vi "Main HMI.vi"() -> ()   [LabVIEW 2020]
uses:
  Control/State - Main HMI.ctl
  Control/Page List Configuration.ctl
  <vilib>/Utility/miscctls.llb/LVRectTypeDef.ctl
  <vilib>/Utility/miscctls.llb/LVPointTypeDef.ctl
  <vilib>/Utility/miscctls.llb/LVPositionTypeDef.ctl
  Control/State - FGV.ctl
  <vilib>/picture/picture.llb/imagedata.ctl
  Control/Header - Page.ctl
  <vilib>/Utility/miscctls.llb/LVBoundsTypeDef.ctl
  Control/State - eFGV.ctl
  Control/Header - User Management.ctl
  Control/Section.ctl
  <vilib>/Platform/browser.llb/Open URL in Default Browser (string).vi
panel:
  out "Project Name":string
  out "Version":string="v1.0"
  in  "Developer":bool
  out "Logo":picture
  in  "Acquire":bool
  out "Log Time":dbl format="%<%H:%M:%S>t"
  in  "Log":bool
  in  "Left":bool caption="1"
  in  "Page":T1(radio)=enum."2"
  in  "Right":bool caption="11"
  in  "Screenshot":bool
  in  "Info":bool
  in  "Alarm Event":bool
  in  "Logout":bool
  in  "Close":bool
  out "Disable":bool
  in  "Error in":errorcluster
  out "Error out":errorcluster
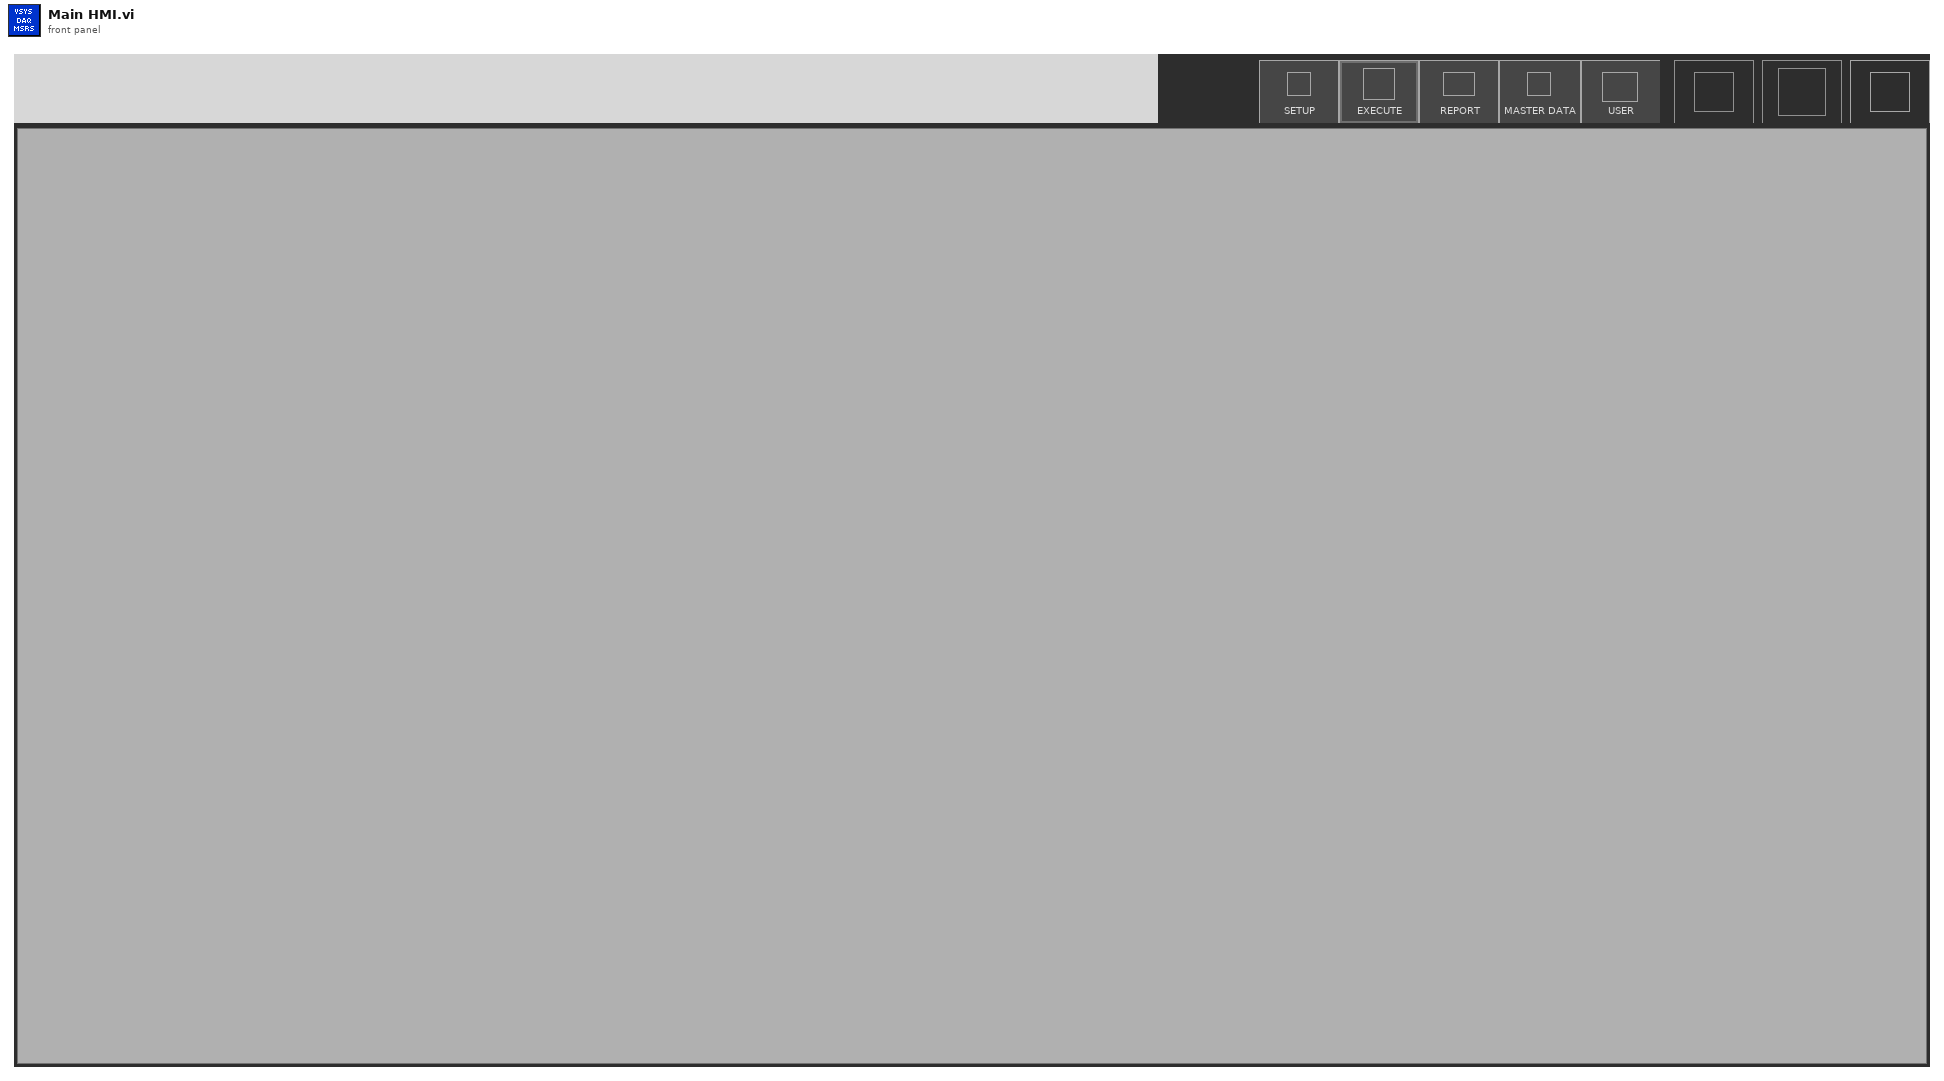
[diagram p1: front panel]
types:
  T1 = enum32{"1", "2", "3", "4", "5", "6", "7", "8", "9", "10", "11", "12", "13", "14", "15"}
  T2 = typedef "Page List Configuration.ctl" = cluster{"HMI Configuration":cluster{"EXE Name":string, "Project Name":string, "Max Page No":i32, "HMI State":enum32{"Invalid", "Standard", "Closed", "Hidden", "Minimized", "Maximized"}, "Version":enum16{"Demo", "User"}, "Check License":bool, "Font Size":u32, "Res: Height":i16, "Res: Width":i16, "License Level":enum16{"Level 1", "Level 2", "Level 3", "Level 4", "Level 5"}, "License Type":enum16{"Free", "Trial", "Subscription", "Perpetual"}}, "All HMI Module":string[], "Default HMI Module":string[], "Page Module":string[], "Page List: Level 1":string[], "Page List: Level 2":string[], "Page List: Level 3":string[], "All RT Module":string[], "Default RT Module":string[], "Acquire Enable Page":string[], "Log Enable Page":string[], "Run Page":string[], "Kill Page":string[], "Button":cluster{"Text":string[], "Tip Strip":string[]}}
  T3 = typedef "LVRectTypeDef.ctl" = cluster{"Left":i16, "Top":i16, "Right":i16, "Bottom":i16}
  T4 = cluster{"Config":T2, "Module":cluster{"Run Module":string[], "Kill Module":string[], "Page Module":string[], "Enable Page":string[]}, "Page Name":string, "T_Out":i32, "Time":timestamp, "Acquire":bool, "Log":bool, "Login":bool, "Discover":bool, "Button Ref":refnum<vi>[], "Direction":string, "Page Size":i32, "Content Area Rect":T3, "Page Size (Hidden)":i32, "Force Logout?":bool, "Update Button":bool, "Event Ref":refnum<event-registration>}
  T5 = typedef "State - Main HMI.ctl" = enum16{"Init", "Init Logo & Name", "Init Size", "Init Page", "Init Button Page", "Init Splitter", "Register Events", "Init Module", "Run Module", "Kill Module", "Change Page", "Update Button Page", "Close Splash Screen", "Idle", "Screenshot", "Developer Mode", "Info", "Move Button Page", "Acquire Event", "Log Event", "Logout", "Check for Exit", "Close"}
  T6 = typedef "LVPositionTypeDef.ctl" = cluster{"Left":i32, "Top":i32}
  T7 = typedef "State - FGV.ctl" = enum16{"Write", "Read"}
  T8 = typedef "imagedata.ctl" = cluster{"image type":i32, "image depth":i32, "image":u8[], "mask":u8[], "colors":u32[], "Rectangle":cluster{"left":i16, "top":i16, "right":i16, "bottom":i16}}
  T9 = enum16{"Init", "Init Module", "Run Module", "Kill Module", "Change Page", "Exit"}
  T10 = typedef "Header - Page.ctl" = enum16{"P1 Main", "P2", "P3 Analysis", "P4 Prediction", "P5 User"}
  T11 = enum8{"Enabled", "Disabled", "Disabled and Grayed Out"}
  T12 = typedef "LVBoundsTypeDef.ctl" = cluster{"Width":u32, "Height":u32}
  T13 = typedef "Header - User Management.ctl" = enum16{"Name", "Staff ID", "Username", "Password", "Access Level", "Status", "Access Page"}
  T14 = enum32{"Invalid", "Standard", "Closed", "Hidden", "Minimized", "Maximized"}
  T15 = enum32{"invalid app kind", "Development System", "Run Time System", "Student Edition", "Embedded LabVIEW", "Evaluation", "Custom"}
  T16 = typedef "Section.ctl" = enum16{"Software Setup", "Config", "Setup", "Network Stream", "MQTT Client", "Setting", "Sample Interval", "Calibration", "Pre-Ranging", "Overrun", "Static", "Filter", "Properties", "Alarm", "Device", "Logging"}
  T17 = typedef "LVPointTypeDef.ctl" = cluster{"Horizontal":i16, "Vertical":i16}
  T18 = typedef "State - eFGV.ctl" = enum16{"Init", "Read", "Write", "Exit"}
  T19 = typedef "License File Parameter.ctl" = cluster{"Expired Time":string, "Computer ID":string, "Product Name":string, "Period":i16, "Activated Time":string, "License Level":enum16{"Level 1", "Level 2", "Level 3", "Level 4", "Level 5"}, "License Type":enum16{"Free", "Trial", "Subscription", "Perpetual"}, "Log Time":string}
  T20 = enum16{"Free", "Trial", "Subscription", "Perpetual"}
  T21 = cluster{"Page Name":string, "All Module":string[], "Default Run Module":string[], "Page Module":string[]}
  T22 = enum16{"Level 1", "Level 2", "Level 3", "Level 4", "Level 5"}
  T23 = enum16{"Pre-Ranging", "Overrun", "Static", "Analysis", "Prediction"}
  T24 = enum32{"Bad", "Idle", "Run top level", "Running"}
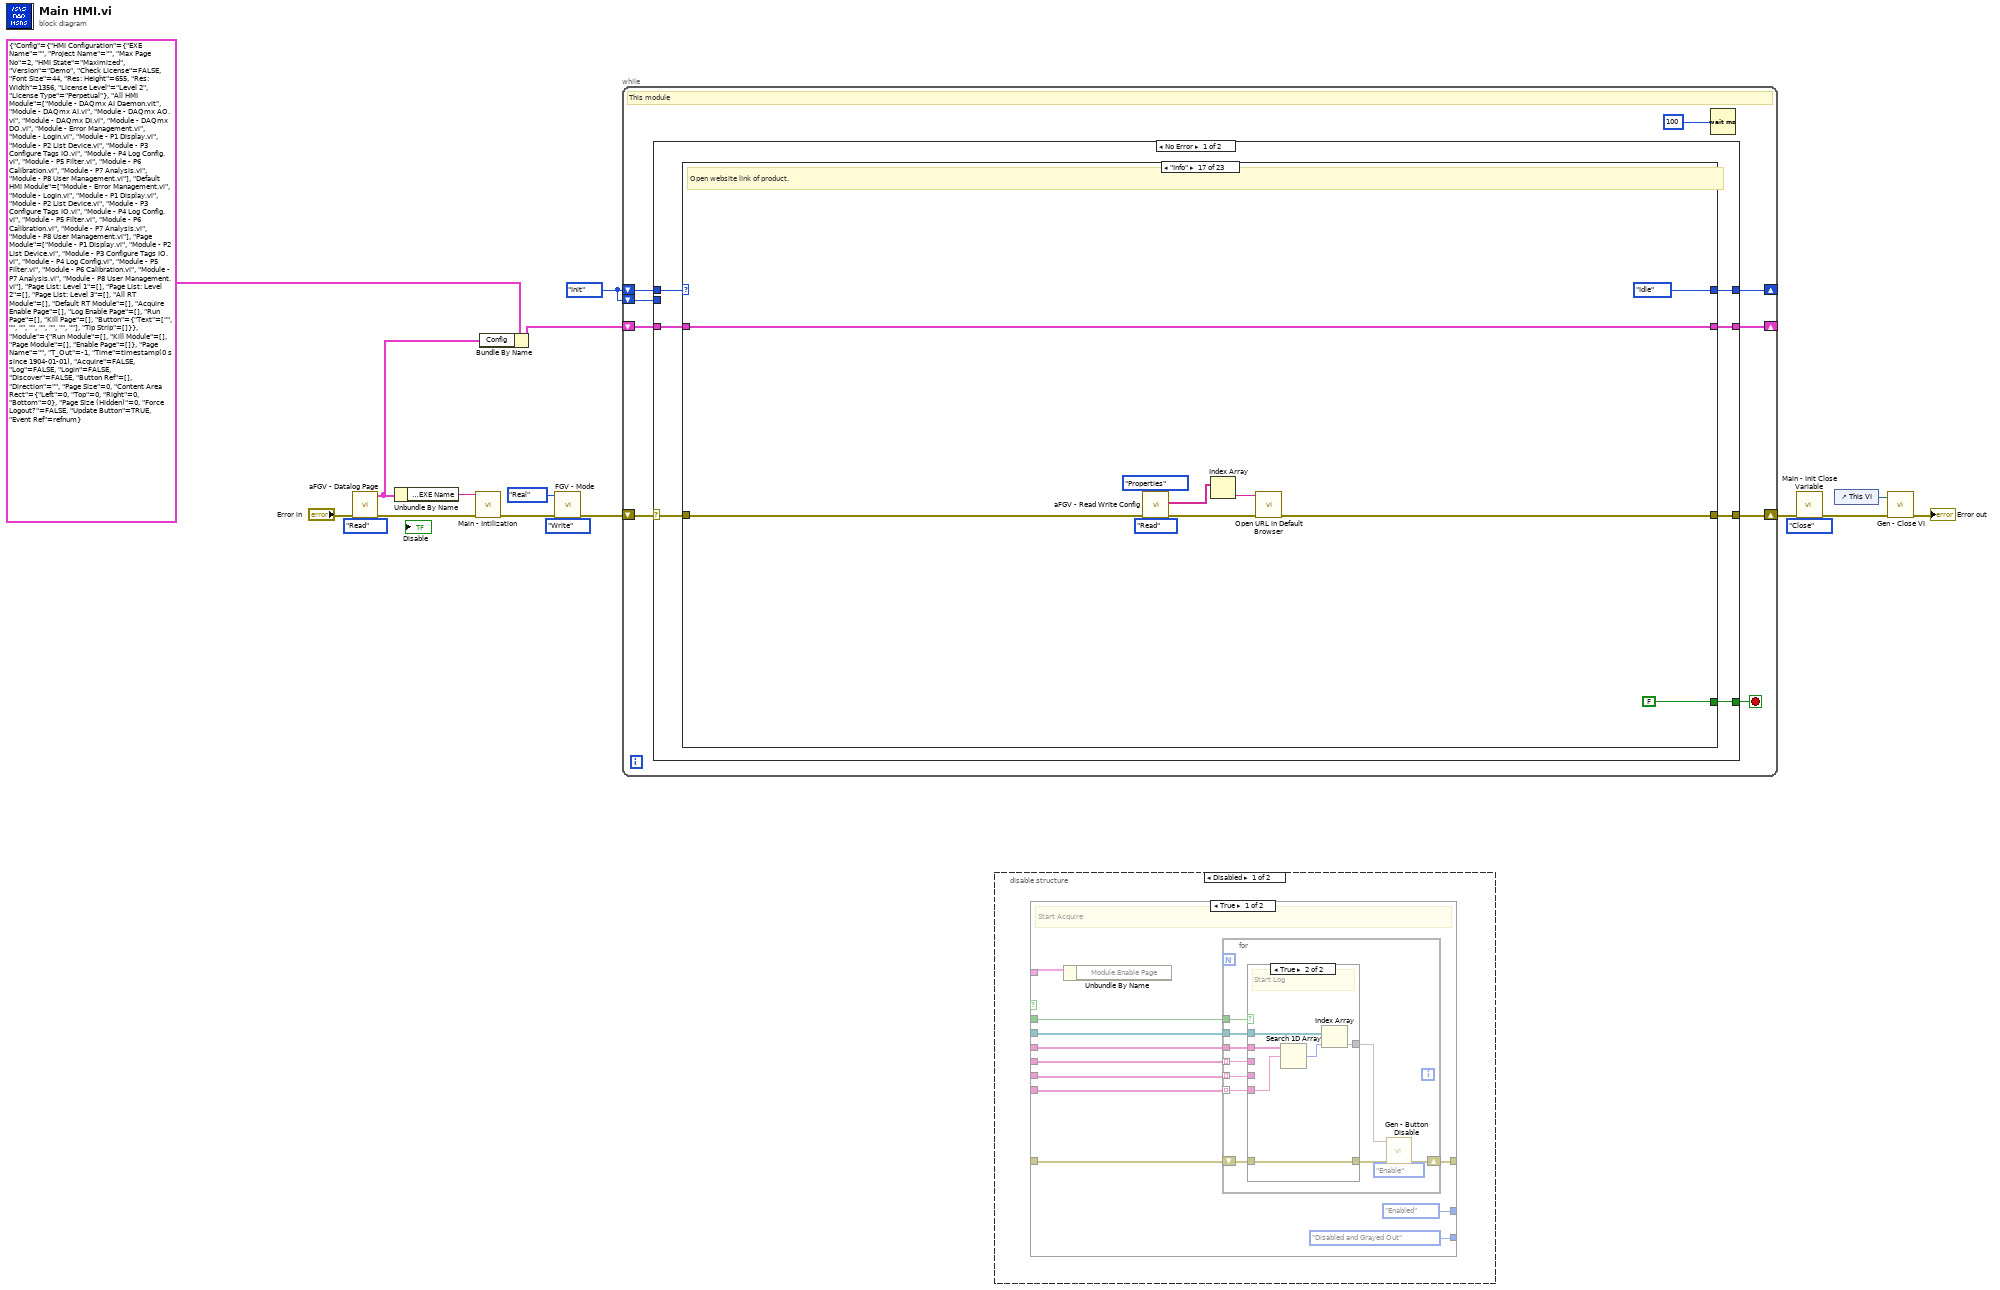
[diagram p0: block diagram]
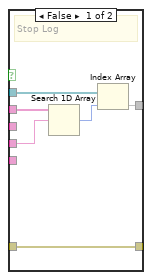
[diagram p2: hidden frame]
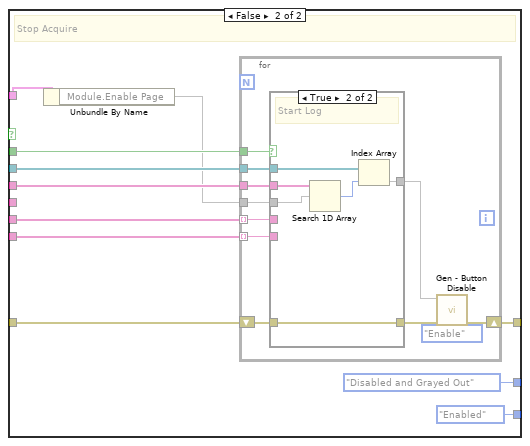
[diagram p3: hidden frame]
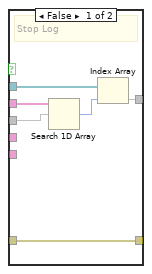
[diagram p4: hidden frame]
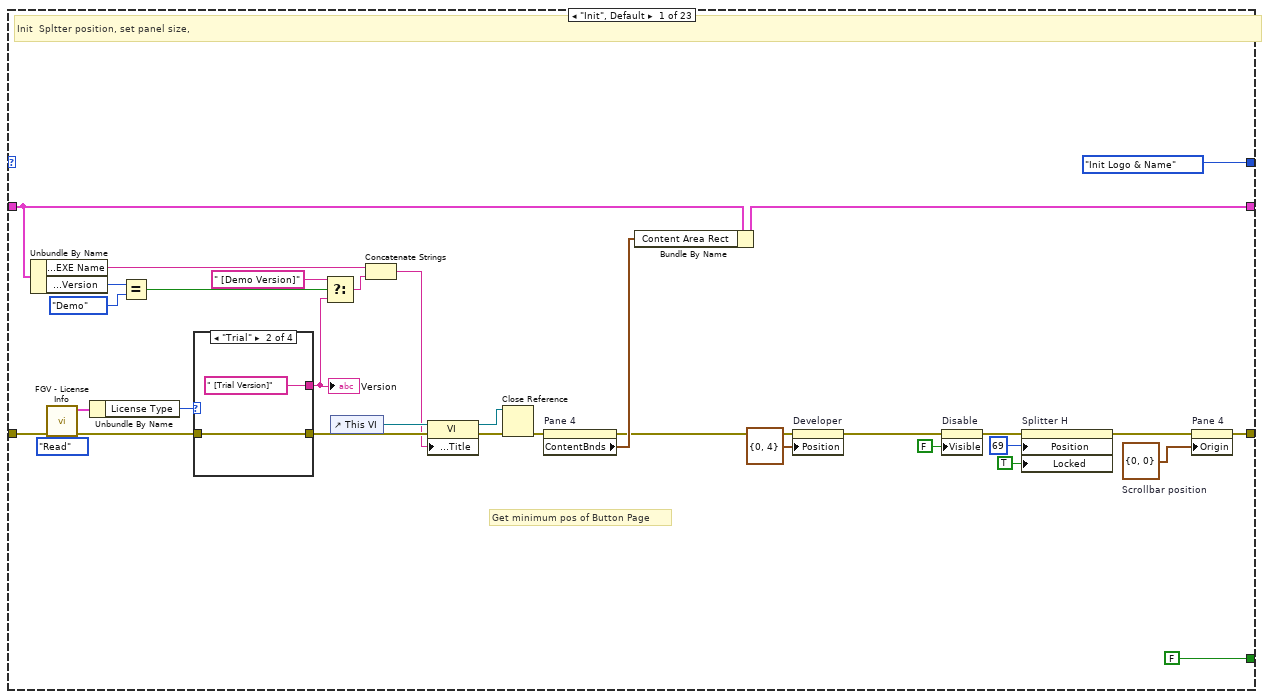
[diagram p6: hidden frame]
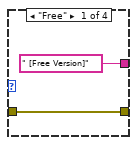
[diagram p7: hidden frame]
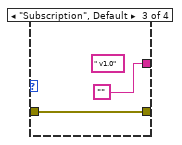
[diagram p8: hidden frame]
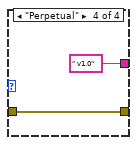
[diagram p9: hidden frame]
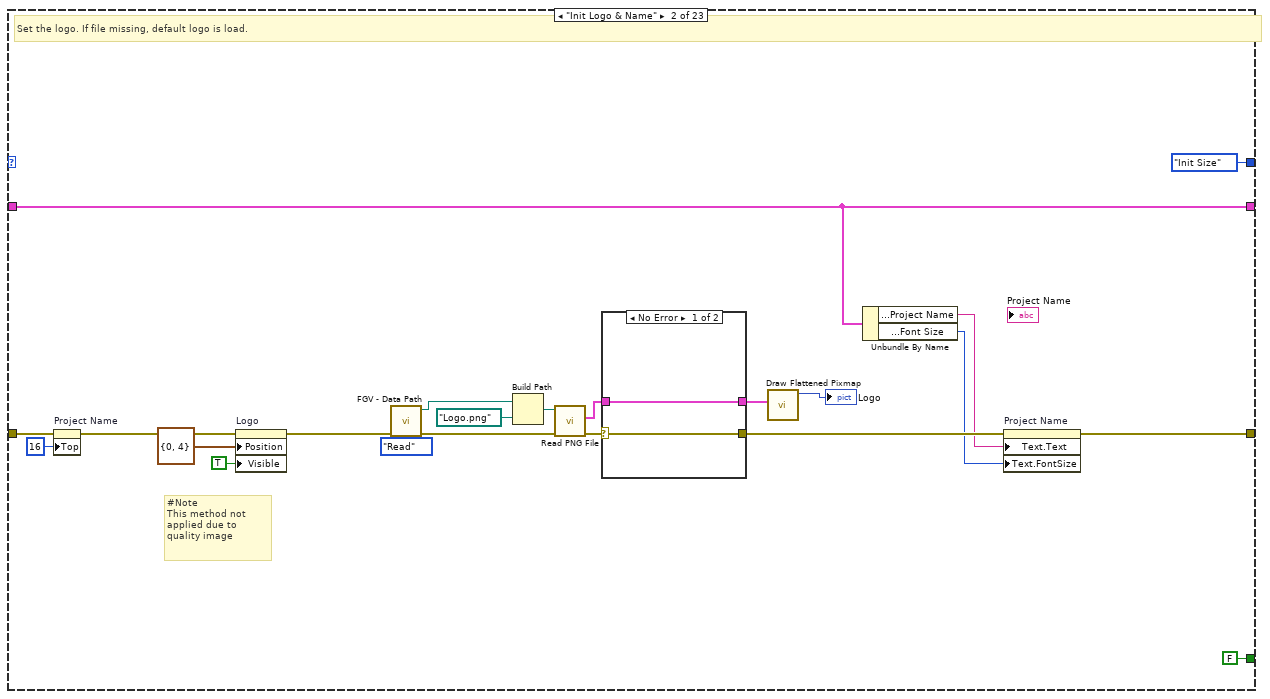
[diagram p10: hidden frame]
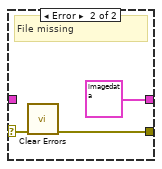
[diagram p11: hidden frame]
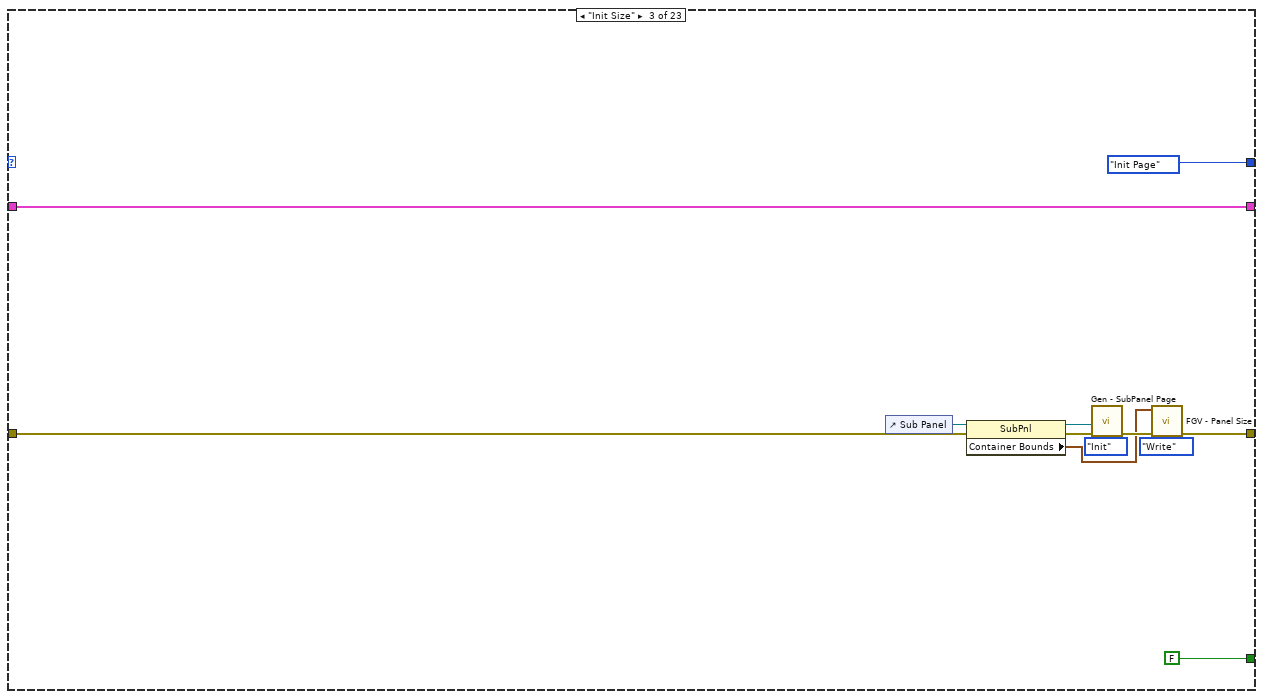
[diagram p12: hidden frame]
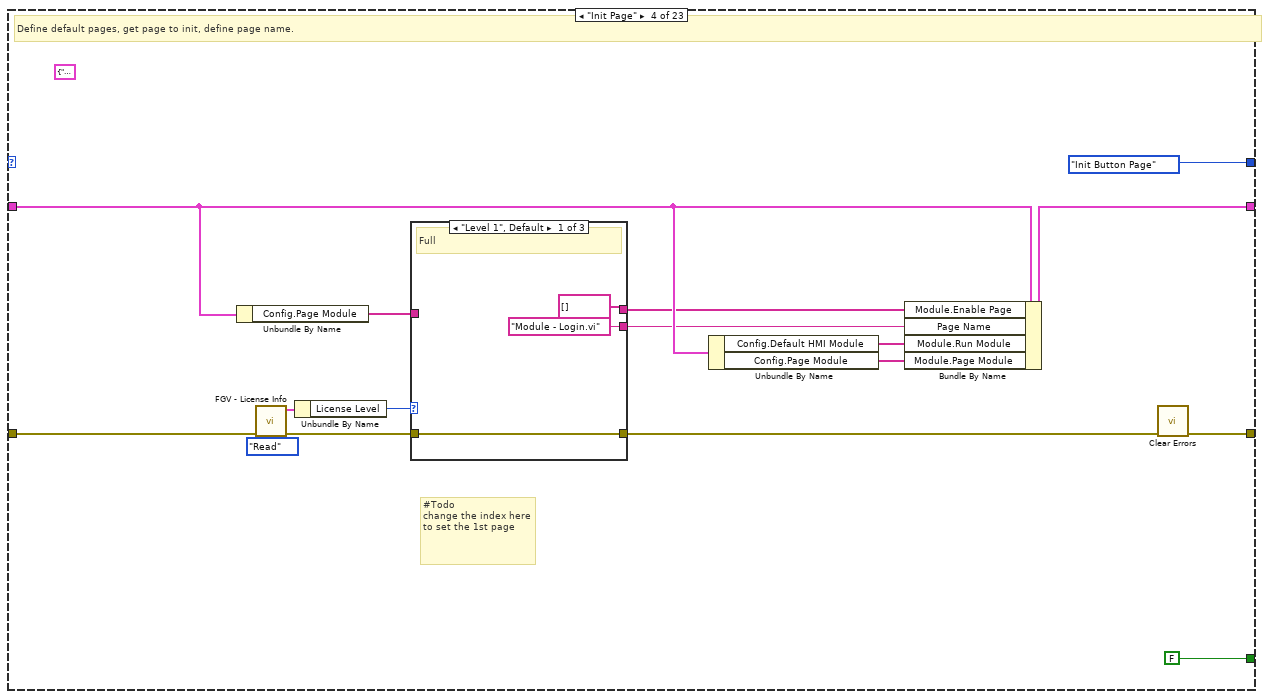
[diagram p13: hidden frame]
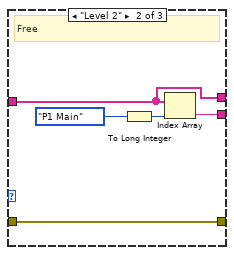
[diagram p14: hidden frame]
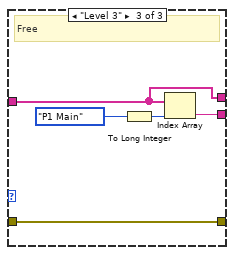
[diagram p15: hidden frame]
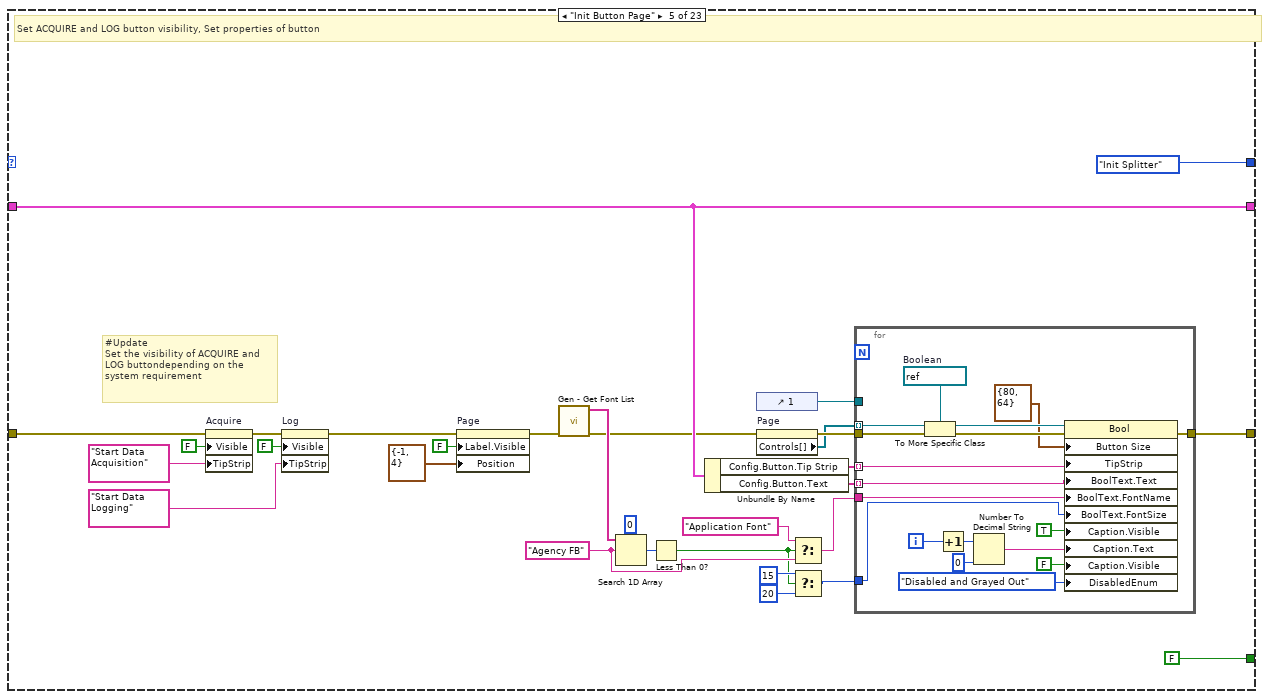
[diagram p16: hidden frame]
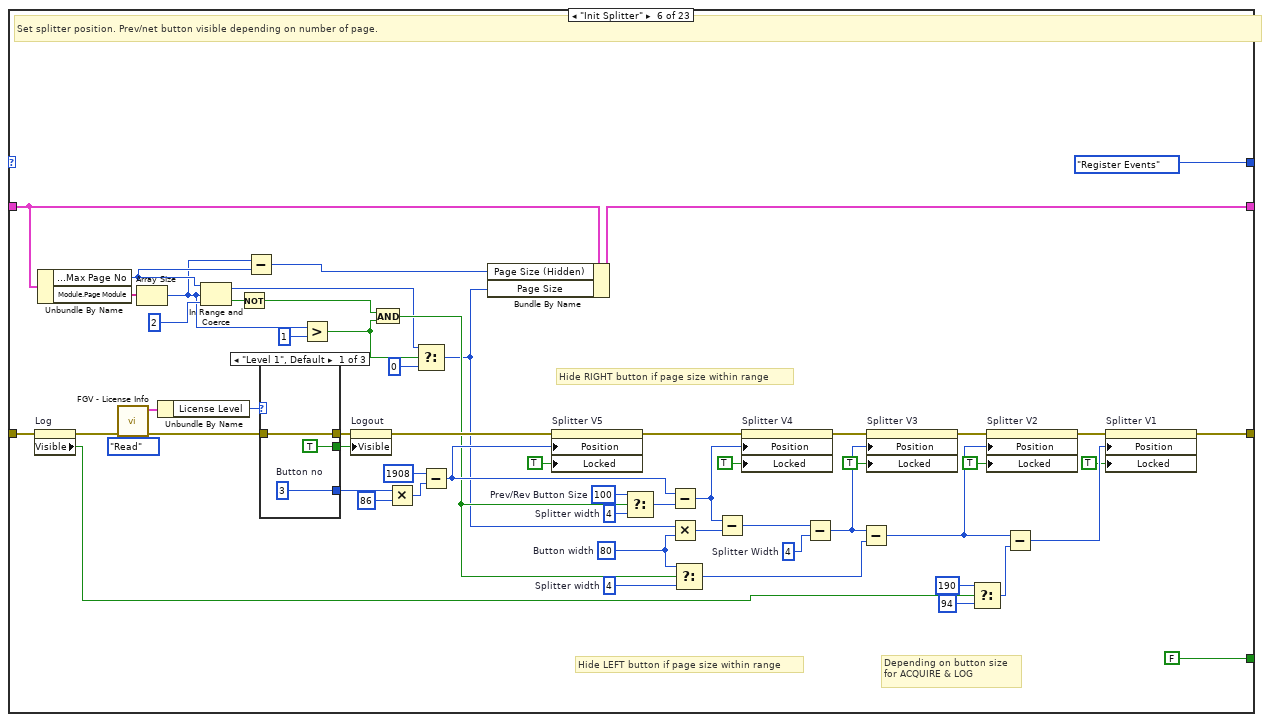
[diagram p17: hidden frame]
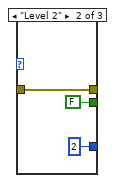
[diagram p18: hidden frame]
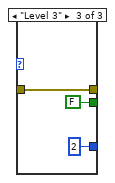
[diagram p19: hidden frame]
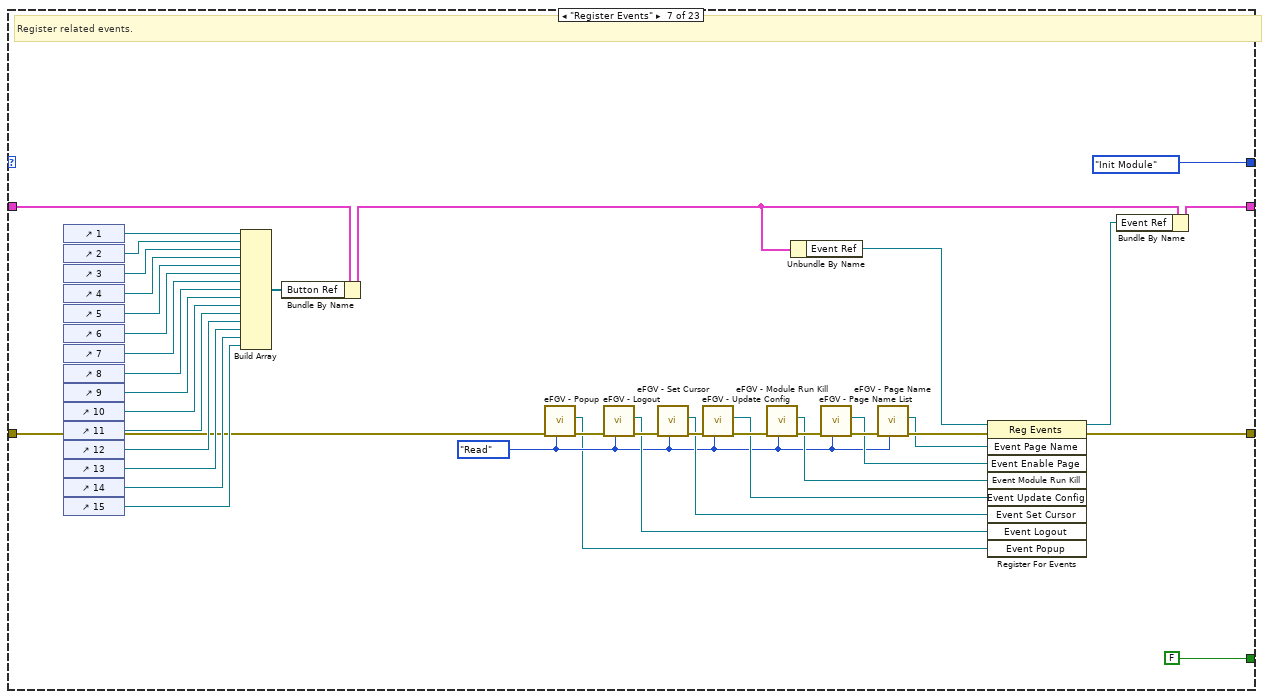
[diagram p20: hidden frame]
diagram:
  w7 = State_-_Main_HMI."Init"
  n1 = call "aFGV - Datalog Page.vi"("Action"=enum16{"Read", "Write"}."Read", "Error In"="Error in") -> ("Error Out"=w4:errorcluster, "Data Out"=w2:T2)  [unwired: 8 in]
  n2 = Unbundle By Name(w2) -> ("HMI Configuration.EXE Name"=w1:string)
  n3 = call "Main - Intilization.vi"("Error In"=w4, "Exe Name"=w1) -> ("Error Out"=w11:errorcluster)  [unwired: 9 in]
  n4 = Bundle By Name(cluster=T4 {"Config"={"HMI Configuration"={"EXE Name"="", "Project Name"="", "Max Page No"=2, "HMI State"=enum."Maximized", "Version"=enum."Demo", "Check License"=FALSE, "Font Size"=44, "Res: Height"=655, "Res: Width"=1356, "License Level"=enum."Level 2", "License Type"=enum."Perpetual"}, "All HMI Module"=["Module - DAQmx AI Daemon.vit", "Module - DAQmx AI.vi", "Module - DAQmx AO.vi", "Module - DAQmx DI.vi", "Module - DAQmx DO.vi", "Module - Error Management.vi", "Module - Login.vi", "Module - P1 Display.vi", "Module - P2 List Device.vi", "Module - P3 Configure Tags IO.vi", "Module - P4 Log Config.vi", "Module - P5 Filter.vi", "Module - P6 Calibration.vi", "Module - P7 Analysis.vi", "Module - P8 User Management.vi"], "Default HMI Module"=["Module - Error Management.vi", "Module - Login.vi", "Module - P1 Display.vi", "Module - P2 List Device.vi", "Module - P3 Configure Tags IO.vi", "Module - P4 Log Config.vi", "Module - P5 Filter.vi", "Module - P6 Calibration.vi", "Module - P7 Analysis.vi", "Module - P8 User Management.vi"], "Page Module"=["Module - P1 Display.vi", "Module - P2 List Device.vi", "Module - P3 Configure Tags IO.vi", "Module - P4 Log Config.vi", "Module - P5 Filter.vi", "Module - P6 Calibration.vi", "Module - P7 Analysis.vi", "Module - P8 User Management.vi"], "Page List: Level 1"=[], "Page List: Level 2"=[], "Page List: Level 3"=[], "All RT Module"=[], "Default RT Module"=[], "Acquire Enable Page"=[], "Log Enable Page"=[], "Run Page"=[], "Kill Page"=[], "Button"={"Text"=["", "", "", "", "", "", "", ""], "Tip Strip"=[]}}, "Module"={"Run Module"=[], "Kill Module"=[], "Page Module"=[], "Enable Page"=[]}, "Page Name"="", "T_Out"=-1, "Time"=timestamp(0 s since 1904-01-01), "Acquire"=FALSE, "Log"=FALSE, "Login"=FALSE, "Discover"=FALSE, "Button Ref"=[], "Direction"="", "Page Size"=0, "Content Area Rect"={"Left"=0, "Top"=0, "Right"=0, "Bottom"=0}, "Page Size (Hidden)"=0, "Force Logout?"=FALSE, "Update Button"=TRUE, "Event Ref"=refnum}, "Config"=w2) -> (w3:T4)
  n5 = call "FGV - Mode.vi"("Action"=enum16{"Read", "Write"}."Write", "Error In"=w11, "Mode in"=enum16{"Sim", "Real"}."Real") -> ("Error Out"=w8:errorcluster)  [unwired: 7 in, 1 out]
  n6 = while {
    shift-right: [w22] -> _
    shift-left: w7 -> [w25]
    shift-right: [w24] -> w15
    shift-left: w8 -> [w26]
    shift-right: [w20] -> _
    shift-left: w3 -> [w21]
    shift-left: w7 -> [w18]
    stop <- w23 stop-if-true
    # "This module"
    n7 = case shown="No Error" w26 {
      selector: w26 -> [w31 w987]
      tunnel: w25 -> [w33 w992]
      tunnel: [w32 w986] -> w24
      tunnel: [w30 FALSE] -> w23
      tunnel: [w29 w992] -> w22
      tunnel: w21 -> [w28 w991]
      tunnel: [w27 w991] -> w20
      tunnel: w18 -> [_ w984]
      frame No Error {
        n8 = case shown="\"Info\"" w33 {
          tunnel: [w58 w77 w103 w121 w169 w241 w292 w304 w311 w318 w346 w373 w495 w507 w652 w681 w729 w742 w781 w812 w868 w910 w954] -> w32
          tunnel: w31 -> [w57 w81 w102 w120 w144 w206 w264 w302 w310 w317 w339 w376 w496 w506 w672 w685 w727 w740 w787 w817 w866 w913 w955]
          tunnel: [FALSE FALSE FALSE FALSE FALSE FALSE FALSE FALSE FALSE FALSE FALSE FALSE FALSE FALSE FALSE FALSE FALSE FALSE FALSE FALSE FALSE FALSE TRUE] -> w30
          tunnel: [State_-_Main_HMI."Init Logo & Name" State_-_Main_HMI."Init Size" State_-_Main_HMI."Init Page" State_-_Main_HMI."Init Button Page" State_-_Main_HMI."Init Splitter" State_-_Main_HMI."Register Events" State_-_Main_HMI."Init Module" State_-_Main_HMI."Run Module" State_-_Main_HMI."Kill Module" State_-_Main_HMI."Change Page" w324 w377 State_-_Main_HMI."Idle" w504 State_-_Main_HMI."Idle" State_-_Main_HMI."Idle" State_-_Main_HMI."Idle" State_-_Main_HMI."Idle" w775 State_-_Main_HMI."Update Button Page" w872 w916 State_-_Main_HMI."Close"] -> w29
          tunnel: w28 -> [w39 w82 w113 w119 w166 w234 w296 w298 w308 w315 w342 w364 w487 w502 w678 w686 w731 w752 w786 w816 w869 w918 w936]
          tunnel: [w64 w82 w113 w127 w166 w225 w258 w298 w308 w315 w329 w364 w487 w499 w678 w686 w731 w752 w774 w814 w870 w918 w936] -> w27
          frame "Init", Default {
            w60 = T17 {"Horizontal"=0, "Vertical"=0}  # Scrollbar position
            # "Get minimum pos of Button Page"
            # "Init  Spltter position, set panel size,"
            n9 = Unbundle By Name(w39) -> ("Config.HMI Configuration.EXE Name"=w37:string, "Config.HMI Configuration.Version"=w38:enum16{"Demo", "User"})
            n10 = call "FGV - License Info.vi"("FGV States"=enum16{"Read", "Write"}."Read", "Error In"=w57) -> ("Error Out"=w53:errorcluster, "License Info"=w55:T19)  [unwired: 8 in]
            n11 = Unbundle By Name(w55) -> ("License Type"=w54:T20)
            n12 = Equal?(x=w38, y=enum16{"Demo", "User"}."Demo") -> (x = y?=w46:bool)
            n13 = case shown="\"Trial\"" w54 {
              tunnel: [w67 w69 w72 w73] -> w48
              tunnel: w53 -> [w67 w69 w72 w73]
              tunnel: [" [Free Version]" ("Version") " [Trial Version]" ("Version") "" " v1.0" ("Version")] -> w45
              frame "Free" {
              }
              frame "Trial" {
              }
              frame "Subscription", Default {
                (unwired) " v1.0" ("Version")
              }
              frame "Perpetual" {
              }
            }
            "Version" <- w45
            n14 = Select(t=" [Demo Version]", s=w46, f=w45) -> (s? t:f=w44:string)
            n15 = control-ref of="This VI"() -> (w52:refnum<vi>)
            n16 = Concatenate Strings(w37, w44) -> (w42:string)
            n17 = property class="VI"(reference=w52, error in=w48, "Front Panel.Title"=w42) -> (reference out=w51:refnum<vi>, error out=w50:errorcluster)
            n18 = Close Reference(reference=w51, error in (no error)=w50) -> (error out=w49:errorcluster)
            n19 = property on="Pane 4" class="Pane"(error in=w49) -> (error out=w36:errorcluster, "ContentBnds"=w63:T3)  [unwired: 1 in, 1 out]
            n20 = Bundle By Name(cluster=w39, "Content Area Rect"=w63) -> (w64:T4)
            n21 = property on="Developer" class="Bool (strict)"(error in=w36, "Position"=T6 {"Left"=0, "Top"=4}) -> (error out=w35:errorcluster)  [unwired: 1 in, 1 out]
            n22 = property on="Disable" class="Bool (strict)"(error in=w35, "Visible"=FALSE) -> (error out=w41:errorcluster)  [unwired: 1 in, 1 out]
            n23 = property on="Splitter H" class="Splitter"(error in=w41, "Position"=69 ("Splitter Position"), "Locked"=TRUE ("Splitter Position Locked")) -> (error out=w59:errorcluster)  [unwired: 1 in, 1 out]
            n24 = property on="Pane 4" class="Pane"(error in=w59, "Origin"=w60) -> (error out=w58:errorcluster)  [unwired: 1 in, 1 out]
          }
          frame "Init Logo & Name" {
            # "#Note\nThis method not applied due to quality image"
            # "Set the logo. If file missing, default logo is load."
            n25 = property on="Project Name" class="Str"(error in=w81, "Top"=16 ("Position:Top")) -> (error out=w80:errorcluster)  [unwired: 1 in, 1 out]
            n26 = property on="Logo" class="Pict"(error in=w80, "Position"=T6 {"Left"=0, "Top"=4}, "Visible"=TRUE) -> (error out=w86:errorcluster)  [unwired: 1 in, 1 out]
            n27 = call "FGV - Data Path.vi"("FGV State"=State_-_FGV."Read", "Error In"=w86) -> ("Error Out"=w89:errorcluster, "Path Out"=w90:path)  [unwired: 8 in]
            n28 = Build Path(base path=w90, name or relative path=path "Logo.png") -> (appended path=w94:path)
            n29 = call <vilib>:"Read PNG File.vi"("error in (no error)"=w89, "path to PNG file"=w94) -> ("error out"=w92:errorcluster, "image data"=w91:T8)  [unwired: 7 in, 1 out]
            n30 = case shown="No Error" w92 {
              selector: w92 -> [w98 w101]
              tunnel: [w98 w99] -> w78
              tunnel: [w97 T8 {"image type"=0, "image depth"=32, "image"=array[57088 elements], "mask"=array[1792 elements], "colors"=[], "Rectangle"={"left"=0, "top"=0, "right"=223, "bottom"=64}} ("image data")] -> w84
              tunnel: w91 -> [w97 _]
              frame No Error {
              }
              frame Error {
                # "File missing"
                n31 = call <vilib>:"Clear Errors.vi"("error in (no error)"=w101) -> ("error out"=w99:errorcluster)  [unwired: 5 in, 1 out]
              }
            }
            n32 = call <vilib>:"Draw Flattened Pixmap.vi"("image data"=w84) -> ("new picture"=→"Logo":picture)  [unwired: 8 in]
            n33 = Unbundle By Name(w82) -> ("Config.HMI Configuration.Project Name"=w76:string, "Config.HMI Configuration.Font Size"=w75:u32)
            n34 = property on="Project Name" class="Str"(error in=w78, "Text.Text"=w76, "Text.FontSize"=w75) -> (error out=w77:errorcluster)  [unwired: 1 in, 1 out]
          }
          frame "Init Size" {
            n35 = control-ref of="Sub Panel"() -> (w110:refnum<vi>)
            n36 = property class="SubPnl"(reference=w110, error in=w102) -> (reference out=w108:refnum<vi>, error out=w109:errorcluster, "Container Bounds"=w106:T12)
            n37 = call "Gen - SubPanel Page.vi"("State"=T9."Init", "Error In"=w109, "Main SubPanel Ref"=w108) -> ("Error Out"=w107:errorcluster)  [unwired: 8 in]
            n38 = call "FGV - Panel Size.vi"("Action"=enum16{"Read", "Write"}."Write", "Error In"=w107, "Size In"=w106) -> ("Error Out"=w103:errorcluster)  [unwired: 7 in, 1 out]
          }
          frame "Init Page" {
            (unwired) T21 {"Page Name"="Module - Login.vi", "All Module"=["Module - DAQmx AI Daemon.vit", "Module - DAQmx AI.vi", "Module - DAQmx AO.vi", "Module - DAQmx DI.vi", "Module - DAQmx DO.vi", "Module - Data Log.vi", "Module - Error Management.vi", "Module - Login.vi", "Module - P1 Display.vi", "Module - P2 List Device.vi", "Module - P3 Configure Tags IO.vi", "Module - P4 Log Config.vi", "Module - P5 Filter.vi", "Module - P6 Calibration.vi", "Module - P7 Analysis.vi", "Module - P8 User Management.vi"], "Default Run Module"=["Module - Error Management.vi", "Module - Login.vi", "Module - P1 Display.vi", "Module - P2 List Device.vi", "Module - P3 Configure Tags IO.vi", "Module - P4 Log Config.vi", "Module - P5 Filter.vi", "Module - P6 Calibration.vi", "Module - P7 Analysis.vi", "Module - P8 User Management.vi"], "Page Module"=["Module - P1 Display.vi", "Module - P2 List Device.vi", "Module - P3 Configure Tags IO.vi", "Module - P4 Log Config.vi", "Module - P5 Filter.vi", "Module - P6 Calibration.vi", "Module - P7 Analysis.vi", "Module - P8 User Management.vi"]}
            # "#Todo \nchange the index here to set the 1st page"
            # "Define default pages, get page to init, define page name."
            n39 = Unbundle By Name(w119) -> ("Config.Page Module"=w117:string[])
            n40 = call "FGV - License Info.vi"("FGV States"=enum16{"Read", "Write"}."Read", "Error In"=w120) -> ("Error Out"=w123:errorcluster, "License Info"=w125:T19)  [unwired: 8 in]
            n41 = Unbundle By Name(w125) -> ("License Level"=w122:T22)
            n42 = case shown="\"Level 1\", Default" w122 {
              tunnel: [w132 w137 w142] -> w124
              tunnel: w123 -> [w132 w137 w142]
              tunnel: w117 -> [_ w133 w138]
              tunnel: ["Module - Login.vi" ("String") w135 w140] -> w116
              tunnel: [string[] [] ("Page Module") w133 w138] -> w115
              frame "Level 1", Default {
                # "Full"
              }
              frame "Level 2" {
                # "Free"
                n43 = To Long Integer(number=Header_-_Page."P1 Main" ("Header - Page")) -> (32bit integer=w134:i32)
                n44 = Index Array(array=w133, index=w134) -> (element=w135:string)
              }
              frame "Level 3" {
                # "Free"
                n45 = To Long Integer(number=Header_-_Page."P1 Main" ("Header - Page")) -> (32bit integer=w139:i32)
                n46 = Index Array(array=w138, index=w139) -> (element=w140:string)
              }
            }
            n47 = Unbundle By Name(w119) -> ("Config.Default HMI Module"=w118:string[], "Config.Page Module"=w114:string[])
            n48 = Bundle By Name(cluster=w119, "Module.Enable Page"=w115, "Page Name"=w116, "Module.Run Module"=w118, "Module.Page Module"=w114) -> (w127:T4)
            n49 = call <vilib>:"Clear Errors.vi"("error in (no error)"=w124) -> ("error out"=w121:errorcluster)  [unwired: 5 in, 1 out]
          }
          frame "Init Button Page" {
            (unwired) 0 ("y")
            w161 = "Agency FB" ("Boolean Text.Font:Name")
            # "#Update\nSet the visibility of ACQUIRE and LOG buttondepending on the system requirement"
            # "Set ACQUIRE and LOG button visibility, Set properties of button"
            n50 = property on="Acquire" class="Bool (strict)"(error in=w144, "Visible"=FALSE, "TipStrip"="Start Data Acquisition" ("Tip Strip")) -> (error out=w149:errorcluster)  [unwired: 1 in, 1 out]
            n51 = property on="Log" class="Bool (strict)"(error in=w149, "Visible"=FALSE, "TipStrip"="Start Data Logging" ("Tip Strip")) -> (error out=w143:errorcluster)  [unwired: 1 in, 1 out]
            n52 = property on="Page" class="RadioBtnsControl (strict)"(error in=w143, "Label.Visible"=FALSE, "Position"=T6 {"Left"=-1, "Top"=4}) -> (error out=w151:errorcluster)  [unwired: 1 in, 1 out]
            n53 = call "Gen - Get Font List.vi"("Error In"=w151) -> ("Error Out"=w154:errorcluster, "Font List"=w155:string[])  [unwired: 9 in]
            n54 = Search 1D Array(1D array=w155, element=w161) -> (index of element=w163:i32)  [unwired: 1 in]
            n55 = Less Than 0?(x=w163) -> (x < 0?=w157:bool)
            n56 = Unbundle By Name(w166) -> ("Config.Button.Tip Strip"=w150:string[], "Config.Button.Text"=w165:string[])
            n57 = control-ref of="1"() -> (w167:refnum<vi>)
            n58 = property on="Page" class="RadioBtnsControl (strict)"(error in=w154) -> (error out=w168:errorcluster, "Controls[]"=w164:refnum<vi>[])  [unwired: 1 in, 1 out]
            n59 = Select(t="Application Font" ("Boolean Text.Font:Name"), s=w157, f=w161) -> (s? t:f=w160:string)
            n60 = Select(t=u32 15 ("Boolean Text.Font:Size"), s=w157, f=u32 20) -> (s? t:f=w158:u32)
            n61 = for {
              tunnel: [w189] -> w169
              tunnel: w168 -> [w182]
              tunnel: w164 -> [w184] mode=indexing
              tunnel: w167 -> [_]
              tunnel: w165 -> [w173] mode=indexing
              tunnel: w160 -> [w176]
              tunnel: w158 -> [w175]
              tunnel: w150 -> [w172] mode=indexing
              i -> [w187]
              w174 = refnum<vi> refnum  # Boolean
              n62 = To More Specific Class(target class=w174, reference=w184, error in=w182) -> (specific class reference=w185:refnum<vi>, error out=w183:errorcluster)
              n63 = Increment(x=w187) -> (x+1=w188:i32)
              n64 = Number To Decimal String(number=w188, width (-)=i16 0) -> (decimal integer string=w181:string)
              n65 = property class="Bool"(reference=w185, error in=w183, "Button Size"=T12 {"Width"=80, "Height"=64}, "TipStrip"=w172, "BoolText.Text"=w173, "BoolText.FontName"=w176, "BoolText.FontSize"=w175, "Caption.Visible"=TRUE, "Caption.Text"=w181, "Caption.Visible"=FALSE, "DisabledEnum"=T11."Disabled and Grayed Out" ("Disabled")) -> (error out=w189:errorcluster)  [unwired: 1 out]
            }
          }
          frame "Init Splitter" {
            w224 = 80  # Button width
            w227 = 4  # Splitter width
            w230 = 4  # Splitter width
            w232 = 100  # Prev/Rev Button Size
            w236 = 4  # Splitter Width
            # "Depending on button size for ACQUIRE & LOG"
            # "Hide LEFT button if page size within range"
            # "Hide RIGHT button if page size within range"
            # "Set splitter position. Prev/net button visible depending on number of page."
            n66 = property on="Log" class="Bool (strict)"(error in=w206) -> (error out=w205:errorcluster, "Visible"=w204:bool)  [unwired: 1 in, 1 out]
            n67 = Unbundle By Name(w234) -> ("Config.HMI Configuration.Max Page No"=w199:i32, "Module.Page Module"=w233:string[])
            n68 = call "FGV - License Info.vi"("FGV States"=enum16{"Read", "Write"}."Read", "Error In"=w205) -> ("Error Out"=w222:errorcluster, "License Info"=w221:T19)  [unwired: 8 in]
            n69 = Array Size(array=w233) -> (size(s)=w197:i32)
            n70 = Unbundle By Name(w221) -> ("License Level"=w223:T22)
            n71 = In Range and Coerce(upper limit=w199, x=w197, lower limit=2 ("HMI Configuration.Max Page No")) -> (coerced(x)=w191:i32, In Range?=w228:bool)
            n72 = Not(x=w228) -> (.not. x?=w195:bool)
            n73 = Subtract(x=w197, y=w199) -> (x-y=w198:i32)
            n74 = case shown="\"Level 1\", Default" w223 {
              tunnel: [w250 w253 w256] -> w218
              tunnel: w222 -> [w250 w253 w256]
              tunnel: [TRUE ("Visible") FALSE ("Visible") FALSE ("Visible")] -> w217
              tunnel: [w248 2 ("Button no") 2 ("Button no")] -> w207
              frame "Level 1", Default {
                w248 = 3  # Button no
              }
              frame "Level 2" {
              }
              frame "Level 3" {
              }
            }
            n75 = Greater?(x=w197, y=1) -> (0:w193:bool)
            n76 = property on="Logout" class="Bool"(error in=w218, "Visible"=w217) -> (error out=w219:errorcluster)  [unwired: 1 in, 1 out]
            n77 = And(x=w195, y=w193) -> (x .and. y?=w194:bool)
            n78 = Multiply(x=w207, y=86) -> (x*y=w208:i32)
            n79 = Select(t=w191, s=w193, f=0) -> (s? t:f=w190:i32)
            n80 = Subtract(x=1908 ("Splitter Position"), y=w208) -> (x-y=w209:i32)
            n81 = Bundle By Name(cluster=w234, "Page Size (Hidden)"=w198, "Page Size"=w190) -> (w225:T4)
            n82 = property on="Splitter V5" class="Splitter"(error in=w219, "Position"=w209, "Locked"=TRUE ("Splitter Position Locked")) -> (error out=w235:errorcluster)  [unwired: 1 in, 1 out]
            n83 = Select(t=w232, s=w194, f=w230) -> (s? t:f=w231:i32)
            n84 = Subtract(x=w209, y=w231) -> (x-y=w229:i32)
            n85 = Multiply(x=w190, y=w224) -> (x*y=w243:i32)
            n86 = Select(t=w224, s=w194, f=w227) -> (s? t:f=w226:i32)
            n87 = Subtract(x=w229, y=w243) -> (x-y=w238:i32)
            n88 = property on="Splitter V4" class="Splitter"(error in=w235, "Position"=w229, "Locked"=TRUE ("Splitter Position Locked")) -> (error out=w244:errorcluster)  [unwired: 1 in, 1 out]
            n89 = Subtract(x=w238, y=w236) -> (x-y=w237:i32)
            n90 = Subtract(x=w237, y=w226) -> (x-y=w240:i32)
            n91 = property on="Splitter V3" class="Splitter"(error in=w244, "Position"=w237, "Locked"=TRUE ("Splitter Position Locked")) -> (error out=w245:errorcluster)  [unwired: 1 in, 1 out]
            n92 = Select(t=190 ("y"), s=w204, f=94 ("y")) -> (s? t:f=w202:i32)
            n93 = property on="Splitter V2" class="Splitter"(error in=w245, "Position"=w240, "Locked"=TRUE ("Splitter Position Locked")) -> (error out=w242:errorcluster)  [unwired: 1 in, 1 out]
            n94 = Subtract(x=w240, y=w202) -> (x-y=w239:i32)
            n95 = property on="Splitter V1" class="Splitter"(error in=w242, "Position"=w239, "Locked"=TRUE ("Splitter Position Locked")) -> (error out=w241:errorcluster)  [unwired: 1 in, 1 out]
          }
          frame "Register Events" {
            w262 = State_-_eFGV."Read" ("FGV State")
            # "Register related events."
            n96 = control-ref of="1"() -> (w288:refnum<vi>)
            n97 = control-ref of="2"() -> (w287:refnum<vi>)
            n98 = control-ref of="3"() -> (w286:refnum<vi>)
            n99 = control-ref of="4"() -> (w285:refnum<vi>)
            n100 = control-ref of="5"() -> (w284:refnum<vi>)
            n101 = control-ref of="6"() -> (w283:refnum<vi>)
            n102 = control-ref of="7"() -> (w282:refnum<vi>)
            n103 = control-ref of="8"() -> (w277:refnum<vi>)
            n104 = control-ref of="9"() -> (w275:refnum<vi>)
            n105 = control-ref of="10"() -> (w274:refnum<vi>)
            n106 = control-ref of="11"() -> (w273:refnum<vi>)
            n107 = control-ref of="12"() -> (w272:refnum<vi>)
            n108 = control-ref of="13"() -> (w271:refnum<vi>)
            n109 = control-ref of="14"() -> (w270:refnum<vi>)
            n110 = control-ref of="15"() -> (w269:refnum<vi>)
            n111 = Build Array(w288, w287, w286, w285, w284, w283, w282, w277, w275, w274, w273, w272, w271, w270, w269) -> (w276:refnum<vi>[])
            n112 = Bundle By Name(cluster=w296, "Button Ref"=w276) -> (w260:T4)
            n113 = call "eFGV - Popup.vi"("Action"=w262, "Error In"=w264) -> ("Error Out"=w263:errorcluster, "Event Popup"=w261:refnum<user-event>)  [unwired: 7 in, 1 out]
            n114 = call "eFGV - Logout.vi"("Action"=w262, "Error In"=w263) -> ("Error Out"=w266:errorcluster, "Event Logout"=w265:refnum<user-event>)  [unwired: 7 in, 1 out]
            n115 = call "eFGV - Set Cursor.vi"("FGV State"=w262, "Error In"=w266) -> ("Error Out"=w268:errorcluster, "Event Set Cursor"=w267:refnum<user-event>)  [unwired: 7 in, 1 out]
            n116 = call "eFGV - Update Config.vi"("Action"=w262, "Error In"=w268) -> ("Error Out"=w279:errorcluster, "Event Update Config"=w278:refnum<user-event>)  [unwired: 7 in, 1 out]
            n117 = call "eFGV - Module Run Kill.vi"("Action"=w262, "Error In"=w279) -> ("Error Out"=w281:errorcluster, "Event Module Run Kill"=w280:refnum<user-event>)  [unwired: 7 in, 1 out]
            n118 = Unbundle By Name(w260) -> ("Event Ref"=w259:refnum<event-registration>)
            n119 = call "eFGV - Page Name List.vi"("Action"=w262, "Error In"=w281) -> ("Error Out"=w290:errorcluster, "Event Enable Page"=w289:refnum<user-event>)  [unwired: 7 in, 1 out]
            n120 = call "eFGV - Page Name.vi"("Action"=w262, "Error In"=w290) -> ("Error Out"=w293:errorcluster, "Event Page Name"=w291:refnum<user-event>)  [unwired: 7 in, 1 out]
            n121 = register-events(reference=w259, error in=w293, w291, w289, w280, w278, w267, w265, w261) -> (reference out=w257:refnum<event-registration>, error out=w292:errorcluster)
            n122 = Bundle By Name(cluster=w260, "Event Ref"=w257) -> (w258:T4)
          }
          frame "Init Module" {
            # "Init and run all listed module. If module is running, it will abort  and then run the module."
            n123 = Unbundle By Name(w298) -> ("Config.All HMI Module"=w297:string[])
            n124 = call "FGV - Module Path.vi"("FGV State"=State_-_FGV."Read", "Error In"=w302) -> ("Error Out"=w299:errorcluster, "Path Out"=w300:path)  [unwired: 8 in]
            n125 = call "Gen - SubPanel Page.vi"("State"=T9."Init Module", "Error In"=w299, "Module List"=w297, "Path to Modules Folder"=w300) -> ("Error Out"=w304:errorcluster)  [unwired: 7 in]
          }
          frame "Run Module" {
            # "Init and run all listed module. If module is running, it will abort  and then run the module."
            n126 = Unbundle By Name(w308) -> ("Module.Run Module"=w307:string[])
            n127 = call "Gen - SubPanel Page.vi"("State"=T9."Run Module", "Error In"=w310, "Module List"=w307) -> ("Error Out"=w311:errorcluster)  [unwired: 8 in]
          }
          frame "Kill Module" {
            # "Init and run all listed module. If module is running, it will abort  and then run the module."
            n128 = Unbundle By Name(w315) -> ("Module.Kill Module"=w314:string[])
            n129 = call "Gen - SubPanel Page.vi"("State"=T9."Kill Module", "Error In"=w317, "Module List"=w314) -> ("Error Out"=w318:errorcluster)  [unwired: 8 in]
          }
          frame "Change Page" {
            # "Change to selected page."
            n130 = Unbundle By Name(w342) -> ("Module.Page Module"=w340:string[], "Page Name"=w336:string)
            n131 = Search 1D Array(1D array=w340, element=w336) -> (index of element=w338:i32)  [unwired: 1 in]
            n132 = Less Than 0?(x=w338) -> (x < 0?=w337:bool)
            n133 = case shown="True" w337 {
              tunnel: w339 -> [w349 w359]
              tunnel: [w349 w358] -> w335
              tunnel: w338 -> [w348 _]
              tunnel: [w348 w351] -> w332
              frame False {
              }
              frame True {
                # "#Todo change the 1st page appeared if required"
                # "Page name not match"
                n134 = call "FGV - Login Status.vi"("Action"=enum16{"Read", "Write"}."Read", "Error In"=w359) -> ("Error Out"=w362:errorcluster, "Username Out"=w363:string)  [unwired: 7 in, 1 out]
                n135 = call "User - Get Info.vi"("Info State"=Header_-_User_Management."Access Level", "Error In"=w362, "Username:"=w363) -> ("Error Out"=w358:errorcluster, "Data Out"=w357:string)  [unwired: 7 in]
                n136 = Not Equal?(x="Admin", y=w357) -> (x != y?=w353:bool)
                n137 = Select(t=Header_-_Page."P5 User", s=w353, f=Header_-_Page."P1 Main") -> (s? t:f=w352:T10)
                n138 = Type Cast(type=0 ("index of element"), x=w352) -> (*(type *) &x=w351:i32)
              }
            }
            n139 = Type Cast(type=T1."1" ("Page"), x=w332) -> (*(type *) &x=w333:T1)
            n140 = Unbundle By Name(w342) -> ("Update Button"=w322:bool, "Acquire"=w323:bool, "Page Name"=w321:string)
            n141 = First Call?() -> (First Call?: T/F=w344:bool)
            n142 = property on="Page" class="RadioBtnsControl (strict)"(error in=w335, "Value"=w333) -> (error out=w334:errorcluster)  [unwired: 1 in, 1 out]
            n143 = call "Gen - SubPanel Page.vi"("State"=T9."Change Page", "Module Name"=w321, "Error In"=w334) -> ("Error Out"=w346:errorcluster)  [unwired: 8 in]
            n144 = Select(t=State_-_Main_HMI."Close Splash Screen", s=w344, f=State_-_Main_HMI."Update Button Page") -> (s? t:f=w327:T5)
            n145 = Select(t=State_-_Main_HMI."Update Button Page", s=w322, f=State_-_Main_HMI."Idle") -> (s? t:f=w325:T5)
            n146 = Bundle By Name(cluster=w342, "Update Button"=TRUE) -> (w329:T4)
            n147 = Select(t=w327, s=w323, f=w325) -> (s? t:f=w324:T5)
          }
          frame "Update Button Page" {
            # "Update button depending on current status; login status, access level, discover device, and list of enable page"
            n148 = call "FGV - Login Status.vi"("Action"=enum16{"Read", "Write"}."Read", "Error In"=w376) -> ("Error Out"=w375:errorcluster, "Username Out"=w370:string, "Login?"=w366:bool)  [unwired: 7 in]
            n149 = case shown="True" w366 {
              tunnel: w375 -> [w393 w481]
              tunnel: [w396 w480] -> w369
              tunnel: [w397 T11."Disabled and Grayed Out" ("Disabled")] -> w372
              tunnel: [w395 T11."Disabled and Grayed Out" ("Disabled")] -> w371
              tunnel: w370 -> [w391 _]
              tunnel: [w387 T11."Disabled and Grayed Out" ("Disabled")] -> w365
              tunnel: w364 -> [w382 w476]
              frame True {
                # "If Admin, Acquire button disable"
                # "Login"
                n150 = call "User - Get Info.vi"("Info State"=Header_-_User_Management."Access Level", "Error In"=w393, "Username:"=w391) -> ("Error Out"=w392:errorcluster, "Data Out"=w389:string)  [unwired: 7 in]
                n151 = Unbundle By Name(w382) -> ("Acquire"=w385:bool, "Log"=w384:bool, "Button Ref"=w383:refnum<vi>[])
                n152 = Not Equal?(x=w389, y="Admin") -> (x != y?=w386:bool)
                n153 = for {
                  tunnel: w392 -> [w474]
                  tunnel: [w473] -> w394
                  tunnel: w383 -> [w472] mode=indexing
                  n154 = call "Gen - Button Disable.vi"("State"=enum16{"Enable", "Disable", "Disable & Gray"}."Disable & Gray", "Error In"=w474, "Ref in"=w472) -> ("Error Out"=w473:errorcluster)  [unwired: 8 in]
                }
                n155 = case shown="True" w385 {
                  tunnel: [w401 w461] -> w396
                  tunnel: w394 -> [w406 w462]
                  tunnel: w383 -> [w405 _]
                  tunnel: w384 -> [w403 _]
                  tunnel: [T11."Enabled" ("Disabled") T11."Disabled and Grayed Out" ("Disabled")] -> w395
                  tunnel: [T11."Disabled and Grayed Out" ("Disabled") T11."Enabled" ("Disabled")] -> w387
                  tunnel: w382 -> [w400 w458]
                  frame True {
                    # "Start Acquire"
                    n156 = case shown="True" w403 {
                      tunnel: w405 -> [_ _]
                      tunnel: [w411 w435] -> w401
                      tunnel: w406 -> [w412 w436]
                      tunnel: w400 -> [w413 w437]
                      frame False {
                        # "Stop Log"
                        n157 = Unbundle By Name(w413) -> ("Button Ref"=w408:refnum<vi>[], "Module.Page Module"=w409:string[], "Module.Enable Page"=w410:string[], "Config.Acquire Enable Page"=w407:string[])
                        n158 = for {
                          tunnel: w410 -> [w417]
                          tunnel: w409 -> [w419]
                          tunnel: w408 -> [w418]
                          shift-right: [w420] -> w411
                          shift-left: w412 -> [w421]
                          tunnel: w407 -> [w416] mode=indexing
                          n159 = Equal?(x=w417, y=w416) -> (x = y?=w415:bool[])
                          n160 = Or Array Elements(Boolean array=w415) -> (logical OR=w414:bool)
                          n161 = case shown="True" w414 {
                            tunnel: w421 -> [w422 w430]
                            tunnel: [w422 w429] -> w420
                            tunnel: w419 -> [_ w428]
                            tunnel: w418 -> [_ w427]
                            tunnel: w416 -> [_ w426]
                            frame False {
                            }
                            frame True {
                              n162 = Search 1D Array(1D array=w428, element=w426) -> (index of element=w425:i32)  [unwired: 1 in]
                              n163 = Index Array(array=w427, index=w425) -> (element=w423:refnum<vi>)
                              n164 = call "Gen - Button Disable.vi"("State"=enum16{"Enable", "Disable", "Disable & Gray"}."Enable", "Error In"=w430, "Ref in"=w423) -> ("Error Out"=w429:errorcluster)  [unwired: 8 in]
                            }
                          }
                        }
                      }
                      frame True {
                        # "Start Log"
                        n165 = Unbundle By Name(w437) -> ("Button Ref"=w432:refnum<vi>[], "Module.Page Module"=w433:string[], "Module.Enable Page"=w434:string[], "Config.Log Enable Page"=w431:string[])
                        n166 = for {
                          tunnel: w434 -> [w441]
                          tunnel: w433 -> [w443]
                          tunnel: w432 -> [w442]
                          shift-right: [w444] -> w435
                          shift-left: w436 -> [w445]
                          tunnel: w431 -> [w440] mode=indexing
                          n167 = Equal?(x=w441, y=w440) -> (x = y?=w439:bool[])
                          n168 = Or Array Elements(Boolean array=w439) -> (logical OR=w438:bool)
                          n169 = case shown="True" w438 {
                            tunnel: w445 -> [w446 w454]
                            tunnel: [w446 w453] -> w444
                            tunnel: w443 -> [_ w452]
                            tunnel: w442 -> [_ w451]
                            tunnel: w440 -> [_ w450]
                            frame False {
                            }
                            frame True {
                              n170 = Search 1D Array(1D array=w452, element=w450) -> (index of element=w449:i32)  [unwired: 1 in]
                              n171 = Index Array(array=w451, index=w449) -> (element=w447:refnum<vi>)
                              n172 = call "Gen - Button Disable.vi"("State"=enum16{"Enable", "Disable", "Disable & Gray"}."Enable", "Error In"=w454, "Ref in"=w447) -> ("Error Out"=w453:errorcluster)  [unwired: 8 in]
                            }
                          }
                        }
                      }
                    }
                  }
                  frame False {
                    # "Stop Acquire"
                    n173 = Unbundle By Name(w458) -> ("Button Ref"=w456:refnum<vi>[], "Module.Page Module"=w455:string[], "Module.Enable Page"=w457:string[])
                    n174 = for {
                      tunnel: w455 -> [w470]
                      tunnel: w457 -> [w469] mode=indexing
                      tunnel: w456 -> [w467]
                      shift-right: [w466] -> w461
                      shift-left: w462 -> [w468]
                      n175 = Search 1D Array(1D array=w470, element=w469) -> (index of element=w463:i32)  [unwired: 1 in]
                      n176 = Index Array(array=w467, index=w463) -> (element=w465:refnum<vi>)
                      n177 = call "Gen - Button Disable.vi"("State"=enum16{"Enable", "Disable", "Disable & Gray"}."Enable", "Error In"=w468, "Ref in"=w465) -> ("Error Out"=w466:errorcluster)  [unwired: 8 in]
                    }
                  }
                }
                n178 = Select(t=T11."Enabled" ("Disabled"), s=w386, f=T11."Disabled and Grayed Out" ("Disabled")) -> (s? t:f=w397:T11)
              }
              frame False {
                n179 = Unbundle By Name(w476) -> ("Button Ref"=w475:refnum<vi>[])
                n180 = for {
                  tunnel: w481 -> [w484]
                  tunnel: [w483] -> w480
                  tunnel: w475 -> [w485] mode=indexing
                  n181 = call "Gen - Button Disable.vi"("State"=enum16{"Enable", "Disable", "Disable & Gray"}."Disable & Gray", "Error In"=w484, "Ref in"=w485) -> ("Error Out"=w483:errorcluster)  [unwired: 8 in]
                }
              }
            }
            n182 = property on="Log" class="Bool (strict)"(error in=w369, "DisabledEnum"=w371) -> (error out=w368:errorcluster)  [unwired: 1 in, 1 out]
            n183 = First Call?() -> (First Call?: T/F=w380:bool)
            n184 = property on="Acquire" class="Bool (strict)"(error in=w368, "DisabledEnum"=w372) -> (error out=w367:errorcluster)  [unwired: 1 in, 1 out]
            n185 = Select(t=State_-_Main_HMI."Close Splash Screen", s=w380, f=State_-_Main_HMI."Idle") -> (s? t:f=w377:T5)
            n186 = property on="Logout" class="Bool"(error in=w367, "DisabledEnum"=w365) -> (error out=w373:errorcluster)  [unwired: 1 in, 1 out]
          }
          frame "Close Splash Screen" {
            w492 = u8 0  # Transparency
            w493 = TRUE  # Transparently?
            # "This part done one time only. To visible the main  VI after run all listed module. Then  update the FGV - Load Main Status. This FGV will trigger the Splash Screen to close."
            n187 = Unbundle By Name(w487) -> ("Config.HMI Configuration.HMI State"=w486:T14)
            n188 = control-ref of="This VI"() -> (w494:refnum<vi>)
            n189 = call "Gen - VI Transparency.vi"("State"=w486, "Error In"=w496, "Transparency"=w492, "Transparently?"=w493, "Ref VI"=w494) -> ("Error Out"=w491:errorcluster)  [unwired: 5 in, 1 out]
            n190 = call "FGV - Load Main Status.vi"("Action"=enum16{"Read", "Write"}."Write", "Error In"=w491, "Status in"=TRUE) -> ("Error Out"=w495:errorcluster)  [unwired: 7 in, 1 out]
          }
          frame "Idle" {
            n191 = Unbundle By Name(w502) -> ("T_Out"=w501:i32, "Event Ref"=w500:refnum<event-registration>)
            n192 = event shown="[3] \"Developer\": Mouse Down" {
              selector: w500 -> [_ _ _ _ _ _ _ _ _ _ _ _ _ _ _ _ _ _ _ _]
              dyn-events: [_ _ _ _ _ _ _ _ _ _ _ _ _ _ _ _ _ _ _ _] -> w498
              timeout: w501 -> [_ _ _ _ _ _ _ _ _ _ _ _ _ _ _ _ _ _ _ _]
              tunnel: [w513 w516 w518 w541 w553 w563 w569 w584 w589 w592 w595 w597 w602 w608 w613 w618 w624 w629 w637 w644] -> w507
              tunnel: w506 -> [w513 w516 w521 w539 w554 w564 w568 w584 w589 w592 w595 w597 w602 w608 w613 w618 w624 w630 w638 w643]
              tunnel: [State_-_Main_HMI."Idle" State_-_Main_HMI."Screenshot" State_-_Main_HMI."Idle" w545 State_-_Main_HMI."Move Button Page" State_-_Main_HMI."Acquire Event" State_-_Main_HMI."Log Event" State_-_Main_HMI."Change Page" State_-_Main_HMI."Logout" State_-_Main_HMI."Info" State_-_Main_HMI."Check for Exit" ("f") State_-_Main_HMI."Idle" State_-_Main_HMI."Check for Exit" State_-_Main_HMI."Logout" State_-_Main_HMI."Update Button Page" State_-_Main_HMI."Update Button Page" State_-_Main_HMI."Run Module" State_-_Main_HMI."Change Page" State_-_Main_HMI."Idle" State_-_Main_HMI."Idle"] -> w504
              tunnel: [w511 w514 w520 w544 w551 w565 w574 w583 w587 w591 w596 w599 w603 w605 w610 w615 w621 w631 w640 w646] -> w503
              tunnel: w502 -> [w511 w514 w520 w549 w557 w567 w575 w582 w588 w591 w596 w599 w603 w606 w611 w616 w622 w628 w640 w646]
              event Timeout {
                n193 = event-data() -> ()  [unwired: 1 in, 1 out]
                n194 = Unbundle By Name(w511) -> ("Time"=w509:timestamp)
                n195 = Get Date/Time In Seconds() -> (seconds since 1Jan1904=w510:timestamp)
                n196 = Subtract(x=w510, y=w509) -> (x-y=→"Log Time":dbl)
              }
              event "Screenshot": Value Change {
                n197 = event-data() -> ()  [unwired: 1 in, 6 out]
              }
              event "Alarm Event": Mouse Down {
                n198 = event-data() -> ("Mods.Double Click"=w517:bool)  [unwired: 1 in]
                n199 = case shown="True" w517 {
                  tunnel: w521 -> [w522 w526]
                  tunnel: [w522 w528] -> w518
                  frame False {
                  }
                  frame True {
                    n200 = call "FGV - Module Path.vi"("FGV State"=State_-_FGV."Read", "Error In"=w526) -> ("Error Out"=w525:errorcluster, "Path Out"=w523:path)  [unwired: 8 in]
                    n201 = Build Path(base path=w523, name or relative path="Module - Alarm Event.vi") -> (appended path=w531:path)
                    n202 = Open VI Reference(vi path=w531, error in (no error)=w525) -> (vi reference=w535:refnum<vi>, error out=w537:errorcluster)  [unwired: 4 in]
                    n203 = invoke class="VI" method="FP.Open"(reference=w535, error in=w537, "Activate"=TRUE ("Activate?"), "State"=T14."Standard") -> (reference out=w530:refnum<vi>, error out=w536:errorcluster)  [unwired: 1 in, 3 out]
                    n204 = Close Reference(reference=w530, error in (no error)=w536) -> (error out=w529:errorcluster)
                    n205 = property on="Alarm Event" class="Bool"(error in=w529, "Blinking"=FALSE) -> (error out=w528:errorcluster)  [unwired: 1 in, 1 out]
                  }
                }
              }
              event "Developer": Mouse Down {
                n206 = event-data() -> ("Mods.Double Click"=w543:bool)  [unwired: 1 in]
                n207 = Bundle By Name(cluster=w549, "Page Name"="Module - Developer.vi") -> (w544:T4)
                n208 = call "FGV - Login Status.vi"("Action"=enum16{"Read", "Write"}."Read", "Error In"=w539) -> ("Error Out"=w541:errorcluster, "Login?"=w540:bool)  [unwired: 7 in, 1 out]
                n209 = And(x=w543, y=w540) -> (x .and. y?=w542:bool)
                n210 = Select(t=State_-_Main_HMI."Developer Mode", s=w542, f=State_-_Main_HMI."Idle") -> (s? t:f=w545:T5)
              }
              event "Left", "Right": Value Change {
                n211 = event-data() -> ("CtlRef"=w552:refnum<vi>)  [unwired: 1 in]
                n212 = property class="Bool"(reference=w552, error in=w554) -> (reference out=w556:refnum<vi>, error out=w555:errorcluster, "Label.Text"=w550:string)
                n213 = Close Reference(reference=w556, error in (no error)=w555) -> (error out=w553:errorcluster)
                n214 = Bundle By Name(cluster=w557, "Direction"=w550) -> (w551:T4)
              }
              event "Acquire": Value Change {
                n215 = event-data() -> ("NewVal"=w562:bool)  [unwired: 1 in, 5 out]
                n216 = Select(t="Stop Data Acquisition" ("Tip Strip"), s=w562, f="Start Data Acquisition" ("Tip Strip")) -> (s? t:f=w561:string)
                n217 = Bundle By Name(cluster=w567, "Acquire"=w562) -> (w565:T4)
                n218 = property on="Acquire" class="Bool (strict)"(error in=w564, "TipStrip"=w561) -> (error out=w563:errorcluster)  [unwired: 1 in, 1 out]
              }
              event "Log": Value Change {
                n219 = event-data() -> ("NewVal"=w570:bool)  [unwired: 1 in, 5 out]
                n220 = Select(t="Stop Data Logging" ("Tip Strip"), s=w570, f="Start Data Logging" ("Tip Strip")) -> (s? t:f=w571:string)
                n221 = Bundle By Name(cluster=w575, "Log"=w570) -> (w574:T4)
                n222 = property on="Log" class="Bool (strict)"(error in=w568, "TipStrip"=w571) -> (error out=w569:errorcluster)  [unwired: 1 in, 1 out]
              }
              event "Page": Value Change {
                n223 = event-data() -> ("NewVal"=w580:T1)  [unwired: 1 in]
                n224 = Unbundle By Name(w582) -> ("Module.Page Module"=w581:string[])
                n225 = To Long Integer(number=w580) -> (32bit integer=w579:i32)
                n226 = Index Array(array=w581, index=w579) -> (element=w578:string)
                n227 = Bundle By Name(cluster=w582, "Page Name"=w578, "Update Button"=FALSE) -> (w583:T4)
              }
              event "Logout": Value Change {
                n228 = event-data() -> ()  [unwired: 1 in, 6 out]
                n229 = Bundle By Name(cluster=w588, "Force Logout?"=FALSE) -> (w587:T4)
              }
              event "Info": Value Change {
                n230 = event-data() -> ()  [unwired: 1 in, 6 out]
              }
              event "Close": Value Change {
                n231 = event-data() -> ()  [unwired: 1 in, 6 out]
              }
              event Panel Resize {
                n232 = event-data() -> ()  [unwired: 1 in, 8 out]
              }
              event Panel Close? {
                n233 = event-data() -> ()  [unwired: 1 in, 4 out]
                n234 = event-data("Discard?"=TRUE) -> ()  [unwired: 1 in, 1 out]
              }
              event User Event {
                # "Get this event when user update thier username. Force logout required."
                n235 = event-data() -> ()  [unwired: 1 in, 5 out]
                n236 = Bundle By Name(cluster=w606, "Force Logout?"=TRUE) -> (w605:T4)
              }
              event User Event {
                n237 = event-data() -> ("Enable Page"=w609:string[])  [unwired: 1 in]
                n238 = Bundle By Name(cluster=w611, "Module.Enable Page"=w609) -> (w610:T4)
              }
              event User Event {
                (unwired) TRUE ("Discover")
                # "Verified the device is discovered. If false, IO Setting is loaded from file."
                n239 = event-data() -> ("New Config"=w614:bool)  [unwired: 1 in]
                n240 = Bundle By Name(cluster=w616, "Discover"=w614) -> (w615:T4)
              }
              event User Event {
                n241 = event-data() -> ("Run Module"=w620:string[], "Kill Module"=w619:string[])  [unwired: 1 in]
                n242 = Bundle By Name(cluster=w622, "Module.Run Module"=w620, "Module.Kill Module"=w619) -> (w621:T4)
              }
              event User Event {
                # "New page name updated"
                n243 = event-data() -> ("Page Name in"=w626:string)  [unwired: 1 in]
                n244 = Unbundle By Name(w628) -> ("Module.Page Module"=w627:string[])
                n245 = Bundle By Name(cluster=w628, "Page Name"=w626) -> (w631:T4)
                n246 = Search 1D Array(1D array=w627, element=w626) -> (index of element=w625:i32)  [unwired: 1 in]
                n247 = disable-structure shown="Enabled" {
                  disable-tunnel: w630 -> [w635 w636]
                  disable-tunnel: [w634 w636] -> w629
                  disable-tunnel: w625 -> [w633 _]
                  frame Disabled {
                    n248 = property on="Page" class="RadioBtnsControl (strict)"(error in=w635, "Value"=w633) -> (error out=w634:errorcluster)  [unwired: 1 in, 1 out]
                  }
                  frame Enabled {
                  }
                }
              }
              event User Event {
                # "Enable & disable background when popup appeared."
                n249 = event-data() -> ("Popup"=w639:bool)  [unwired: 1 in]
                n250 = property on="Disable" class="Bool (strict)"(error in=w638, "Visible"=w639) -> (error out=w637:errorcluster)  [unwired: 1 in, 1 out]
              }
              event User Event {
                # "Set cursor busy and unset busy"
                n251 = event-data() -> ("Cursor Busy In"=w645:bool)  [unwired: 1 in]
                n252 = case shown="False" w645 {
                  tunnel: [w647 w649] -> w644
                  tunnel: w643 -> [w648 w650]
                  frame False {
                    n253 = call <vilib>:"Unset Busy.vi"("error in (no error)"=w648) -> ("error out"=w647:errorcluster)  [unwired: 10 in]
                  }
                  frame True {
                    n254 = call <vilib>:"Set Busy.vi"("error in (no error)"=w650) -> ("error out"=w649:errorcluster)  [unwired: 9 in, 1 out]
                  }
                }
              }
            }
            n255 = Bundle By Name(cluster=w503, "Event Ref"=w498) -> (w499:T4)
          }
          frame "Screenshot" {
            # "Use to screenshot the whole UI and auto save"
            n256 = control-ref of="This VI"() -> (w673:refnum<vi>)
            n257 = invoke class="VI" method="FP.Get Image"(reference=w673, error in=w672) -> (reference out=w674:refnum<vi>, error out=w675:errorcluster, "image data"=w651:T8)  [unwired: 4 in, 3 out]
            n258 = Close Reference(reference=w674, error in (no error)=w675) -> (error out=w661:errorcluster)
            n259 = call "FGV - Data Path.vi"("FGV State"=State_-_FGV."Read", "Error In"=w661) -> ("Error Out"=w660:errorcluster, "Path Out"=w658:path)  [unwired: 8 in]
            n260 = Get Date/Time In Seconds() -> (seconds since 1Jan1904=w670:timestamp)
            n261 = call "FGV - Data Folder.vi"("Action"=enum16{"Read", "Write"}."Read", "Error In"=w660) -> ("Error Out"=w667:errorcluster, "Mode Out"=w669:T23)  [unwired: 8 in]
            n262 = Format Date/Time String(time format string (%c)="%y%m%d %H%M%S ", seconds (now)=w670) -> (date/time string=w665:string)  [unwired: 1 in]
            n263 = Build Path(base path=w658, name or relative path=path "Data/Screenshot") -> (appended path=w657:path)
            n264 = Format Into String(format string="%s", initial string=w665, error in=w667, w669) -> (resulting string=w664:string, error out=w666:errorcluster)
            n265 = Concatenate Strings(w664, ".png" ("string")) -> (w656:string)
            n266 = Build Path(base path=w657, name or relative path=w656) -> (appended path=w654:path)
            n267 = call <vilib>:"Write PNG File.vi"("error in (no error)"=w666, "image data"=w651, "path to PNG file"=w654) -> ("error out"=w653:errorcluster)  [unwired: 7 in, 1 out]
            n268 = call "Screenshot Flash.vi"("Error In"=w653, "Image Data"=w651) -> ("Error Out"=w652:errorcluster)  [unwired: 8 in, 1 out]
          }
          frame "Developer Mode" {
            # "Run developer page as popup."
            n269 = call "Gen - Get Application Kind.vi"("Error In"=w685) -> ("Error Out"=w684:errorcluster)  [unwired: 9 in, 1 out]
            n270 = case shown="\"Run Time System\"" T15."Run Time System" ("Application:Kind") {
              tunnel: [w717 w720 w722] -> w682
              tunnel: [FALSE ("Login?") w719 TRUE ("Login?")] -> w683
              tunnel: w684 -> [w717 w718 w722]
              frame "invalid app kind", Default {
              }
              frame "Run Time System" {
                n271 = call "Login - Developer Mode.vi"("Error In"=w718) -> ("Error Out"=w720:errorcluster, "Login?"=w719:bool)  [unwired: 9 in]
              }
              frame "Development System" {
              }
            }
            n272 = case shown="True" w683 {
              tunnel: w682 -> [w688 w703]
              tunnel: [w688 w699] -> w681
              frame False {
              }
              frame True {
                n273 = call "FGV - Module Path.vi"("FGV State"=State_-_FGV."Read", "Error In"=w703) -> ("Error Out"=w704:errorcluster, "Path Out"=w701:path)  [unwired: 8 in]
                n274 = Build Path(base path=w701, name or relative path="Module - Developer.vi") -> (appended path=w709:path)
                n275 = Open VI Reference(vi path=w709) -> (vi reference=w708:refnum<vi>)  [unwired: 5 in, 1 out]
                n276 = property class="VI"(reference=w708, error in=w704) -> (reference out=w707:refnum<vi>, error out=w706:errorcluster, "Exec.State"=w705:T24)
                n277 = case shown="\"Run top level\", \"Running\"" w705 {
                  tunnel: w706 -> [w711 w715]
                  tunnel: w707 -> [w710 w714]
                  tunnel: [w710 w712] -> w696
                  tunnel: [w711 w713] -> w691
                  frame Default {
                  }
                  frame "Run top level", "Running" {
                    n278 = invoke class="VI" method="Abort VI"(reference=w714, error in=w715) -> (reference out=w712:refnum<vi>, error out=w713:errorcluster)  [unwired: 1 in, 1 out]
                  }
                }
                n279 = invoke class="VI" method="Run VI"(reference=w696, error in=w691, "Wait until done"=FALSE ("Wait Until Done"), "Auto Dispose Ref"=FALSE ("Auto Dispose Reference")) -> (reference out=w695:refnum<vi>, error out=w694:errorcluster)  [unwired: 1 in, 3 out]
                n280 = invoke class="VI" method="FP.Open"(reference=w695, error in=w694, "Activate"=FALSE ("Activate?"), "State"=T14."Standard") -> (reference out=w693:refnum<vi>, error out=w692:errorcluster)  [unwired: 1 in, 3 out]
                n281 = Close Reference(reference=w693, error in (no error)=w692) -> (error out=w699:errorcluster)
              }
            }
          }
          frame "Info" {
            # "Open website link of product."
            n282 = call "aFGV - Read Write Config.vi"("State"=enum16{"Read", "Write", "Delete"}."Read", "Section"=Section."Properties", "Error In"=w727) -> ("Error Out"=w728:errorcluster, "Data out"=w724:string[])  [unwired: 6 in, 1 out]
            n283 = Index Array(array=w724) -> (element=w723:string)  [unwired: 1 in]
            n284 = call-poly <vilib>:"Open URL in Default Browser.vi"("error in (no error)"=w728, "URL"=w723) -> ("error out"=w729:errorcluster)  [unwired: 4 in, 1 out]
          }
          frame "Move Button Page" {
            w746 = i16 80  # Button Size
            n285 = Unbundle By Name(w752) -> ("Page Size (Hidden)"=w734:i32, "Content Area Rect.Left"=w736:i16, "Direction"=w751:string)
            n286 = property on="Page" class="RadioBtnsControl (strict)"(error in=w740) -> (error out=w739:errorcluster, "Controls[]"=w738:refnum<vi>[])  [unwired: 1 in, 1 out]
            n287 = Array Size(array=w738) -> ()  [unwired: 1 out]
            n288 = To Word Integer(number=w734) -> (16bit integer=w737:i16)
            n289 = Multiply(x=w737, y=w746) -> (x*y=w733:i16)
            n290 = property on="Pane 4" class="Pane"(error in=w739) -> (error out=w749:errorcluster, "Origin"=w750:T17)  [unwired: 1 in, 1 out]
            n291 = Add(x=w733, y=w736) -> ()  [unwired: 1 out]
            n292 = case shown="\"Right\", Default" w751 {
              tunnel: [w758 w762] -> w743
              tunnel: w749 -> [w758 w762]
              tunnel: T17 {"Horizontal"=80, "Vertical"=0} ("y") -> [w757 w761]
              tunnel: w750 -> [w756 w760]
              tunnel: [w755 w759] -> w744
              frame "Left" {
                n293 = Subtract(x=w756, y=w757) -> (x-y=w755:T17)
              }
              frame "Right", Default {
                n294 = Add(x=w760, y=w761) -> (x+y=w759:T17)
              }
            }
            n295 = Unbundle By Name(w744) -> ("Horizontal"=w748:i16)
            n296 = In Range and Coerce(upper limit=w733, x=w748, lower limit=i16 0) -> (coerced(x)=w747:i16)  [unwired: 1 out]
            n297 = Bundle By Name(cluster=w744, "Horizontal"=w747) -> (w741:T17)
            n298 = property on="Pane 4" class="Pane"(error in=w743, "Origin"=w741) -> (error out=w742:errorcluster)  [unwired: 1 in, 1 out]
          }
          frame "Acquire Event" {
            # "#Note\nUse for VSys DAQ. Function remain for other project"
            # "Start acquire. Enable/Disable log button depending on license level. Enable/disable related page."
            n299 = Unbundle By Name(w786) -> ("Acquire"=w785:bool)
            n300 = call "eFGV - Start Acquisition.vi"("FGV State"=State_-_eFGV."Write", "Error In"=w787, "Start Test"=w785) -> ("Error Out"=w784:errorcluster)  [unwired: 6 in, 2 out]
            n301 = case shown="True" w785 {
              selector: w785 -> [w803 _]
              tunnel: [w800 w811] -> w772
              tunnel: w784 -> [w801 w811]
              tunnel: [w805 w810] -> w779
              tunnel: w786 -> [w806 w810]
              tunnel: [T11."Disabled and Grayed Out" ("Disabled") T11."Enabled" ("Disabled")] -> w780
              tunnel: [T11."Enabled" ("Disabled") T11."Disabled and Grayed Out" ("Disabled")] -> w766
              frame False {
                n302 = local write "Log"(w803) -> ()
                n303 = property on="Log Time" class="DigNum (strict)"(error in=w801, "Visible"=w803) -> (error out=w802:errorcluster)  [unwired: 1 in, 1 out]
                n304 = Bundle By Name(cluster=w806, "T_Out"=-1) -> (w805:T4)
                n305 = call "eFGV - Start Log.vi"("Action"=State_-_eFGV."Write", "Error In"=w802, "Start Log"=w803) -> ("Error Out"=w800:errorcluster)  [unwired: 6 in, 2 out]
              }
              frame True {
                # "Start Acquire"
              }
            }
            n306 = property on="Log" class="Bool (strict)"(error in=w772, "DisabledEnum"=w780) -> (error out=w768:errorcluster)  [unwired: 1 in, 1 out]
            n307 = property on="Logout" class="Bool"(error in=w768, "DisabledEnum"=w766) -> (error out=w767:errorcluster)  [unwired: 1 in, 1 out]
            n308 = Unbundle By Name(w779) -> ("Log"=w778:bool, "Config.Page Module"=w764:string[], "Config.Acquire Enable Page"=w763:string[])
            n309 = property on="Page" class="RadioBtnsControl (strict)"(error in=w767) -> (error out=w782:errorcluster, "Controls[]"=w783:refnum<vi>[])  [unwired: 1 in, 1 out]
            n310 = To Long Integer(number=Header_-_Page."P1 Main") -> (32bit integer=w769:i32)
            n311 = for {
              N: 0 -> [_]
              tunnel: w783 -> [w797]
              tunnel: w766 -> [w793]
              tunnel: w764 -> [w792]
              tunnel: w763 -> [w791] mode=indexing
              tunnel: w782 -> [w796]
              tunnel: [w794] -> w781
              n312 = Search 1D Array(1D array=w792, element=w791) -> (index of element=w790:i32)  [unwired: 1 in]
              n313 = Index Array(array=w797, index=w790) -> (element=w795:refnum<vi>)
              n314 = property class="Ctl"(reference=w795, error in=w796, "DisabledEnum"=w793) -> (error out=w794:errorcluster)  [unwired: 1 out]
            }
            n315 = Index Array(array=w764, index=w769) -> (element=w770:string)
            n316 = Bundle By Name(cluster=w779, "Log"=FALSE, "Page Name"=w770) -> (w774:T4)
            n317 = Select(t=State_-_Main_HMI."Log Event", s=w778, f=State_-_Main_HMI."Change Page") -> (s? t:f=w775:T5)
          }
          frame "Log Event" {
            w820 = -1  # T_Out
            w819 = 500  # T_Out
            # "Event when user start/stop data logging. Update eFGV - Start Log and update logging time."
            n318 = Unbundle By Name(w816) -> ("Log"=w815:bool)
            n319 = call "eFGV - Start Log.vi"("Action"=State_-_eFGV."Write", "Error In"=w817, "Start Log"=w815) -> ("Error Out"=w822:errorcluster)  [unwired: 6 in, 2 out]
            n320 = property on="Log Time" class="DigNum (strict)"(error in=w822, "Visible"=w815, "Value"=0.0 ("Log Time")) -> (error out=w821:errorcluster)  [unwired: 1 in, 1 out]
            n321 = Select(t=w819, s=w815, f=w820) -> (s? t:f=w824:i32)
            n322 = disable-structure shown="Disabled" {
              disable-tunnel: w821 -> [w846 w863]
              disable-tunnel: w815 -> [w842 _]
              disable-tunnel: [w841 w863] -> w812
              frame Disabled {
                n323 = property on="Page" class="RadioBtnsControl (strict)"(error in=w846) -> (error out=w847:errorcluster, "Controls[]"=w848:refnum<vi>[])  [unwired: 1 in, 1 out]
                n324 = Select(t=T11."Disabled and Grayed Out" ("Disabled"), s=w842, f=T11."Enabled") -> (s? t:f=w840:T11)
                n325 = for {
                  N: 0 -> [_]
                  tunnel: w848 -> [w862]
                  tunnel: w840 -> [w859]
                  tunnel: i32[] [4, 5, 6] ("index") -> [w858] mode=indexing
                  shift-right: [w857] -> w839
                  shift-left: w847 -> [w861]
                  n326 = Index Array(array=w862, index=w858) -> (element=w860:refnum<vi>)
                  n327 = property class="Ctl"(reference=w860, error in=w861, "DisabledEnum"=w859) -> (error out=w857:errorcluster)  [unwired: 1 out]
                }
                n328 = call "FGV - Login Status.vi"("Action"=enum16{"Read", "Write"}."Read", "Error In"=w839) -> ("Error Out"=w829:errorcluster, "Username Out"=w832:string)  [unwired: 7 in, 1 out]
                n329 = call "User - Get Info.vi"("Info State"=Header_-_User_Management."Access Page", "Error In"=w829, "Username:"=w832) -> ("Error Out"=w828:errorcluster)  [unwired: 7 in, 1 out]
                n330 = call "Gen - System Config.vi"() -> ("Data Out"=w837:T2)  [unwired: 11 in]
                n331 = Unbundle By Name(w837) -> ("Page Module"=w834:string[], "Default RT Run Module"=w833:string[])
                n332 = property on="Page" class="RadioBtnsControl (strict)"(error in=w828) -> (error out=w835:errorcluster, "Controls[]"=w836:refnum<vi>[])  [unwired: 1 in, 1 out]
                n333 = for {
                  N: 0 -> [_]
                  tunnel: w836 -> [w856]
                  tunnel: w840 -> [w852]
                  tunnel: w834 -> [w851]
                  tunnel: w833 -> [w850] mode=indexing
                  tunnel: w835 -> [w855]
                  tunnel: [w853] -> w841
                  n334 = Search 1D Array(1D array=w851, element=w850) -> (index of element=w849:i32)  [unwired: 1 in]
                  n335 = Index Array(array=w856, index=w849) -> (element=w854:refnum<vi>)
                  n336 = property class="Ctl"(reference=w854, error in=w855, "DisabledEnum"=w852) -> (error out=w853:errorcluster)  [unwired: 1 out]
                }
              }
              frame Enabled {
              }
            }
            n337 = Get Date/Time In Seconds() -> (seconds since 1Jan1904=w823:timestamp)
            n338 = Bundle By Name(cluster=w816, "T_Out"=w824, "Time"=w823) -> (w814:T4)
          }
          frame "Logout" {
            n339 = call "eFGV - Start Acquisition.vi"("FGV State"=State_-_eFGV."Read", "Error In"=w866) -> ("Error Out"=w864:errorcluster, "Start Out"=w865:bool)  [unwired: 7 in, 1 out]
            n340 = case shown="False" w865 {
              tunnel: [w880 State_-_Main_HMI."Idle"] -> w872
              tunnel: [w879 w907] -> w870
              tunnel: w869 -> [w874 w907]
              tunnel: [w878 w902] -> w868
              tunnel: w864 -> [w875 w903]
              frame False {
                n341 = Unbundle By Name(w874) -> ("Force Logout?"=w873:bool)
                n342 = case shown="True" w873 {
                  selector: w873 -> [_ w889]
                  tunnel: [w885 w888] -> w877
                  tunnel: [w883 w889] -> w876
                  tunnel: w875 -> [w881 w888]
                  frame False {
                    n343 = call "Gen - Popup Two Button.vi"("Type"=enum16{"Error", "Info"}."Error", "Error in"=w881, "Button text"=string[] ["YES", "NO"], "Message in"="Are you sure to logout?", "Header"="Logout") -> ("Error out"=w885:errorcluster, "Yes?"=w883:bool)  [unwired: 5 in]
                  }
                  frame True {
                  }
                }
                n344 = case shown="True" w876 {
                  tunnel: [State_-_Main_HMI."Idle" State_-_Main_HMI."Change Page"] -> w880
                  tunnel: [w891 w898] -> w879
                  tunnel: w874 -> [w891 w897]
                  tunnel: w877 -> [w890 w893]
                  tunnel: [w890 w896] -> w878
                  frame False {
                  }
                  frame True {
                    n345 = call "FGV - Login Status.vi"("Action"=enum16{"Read", "Write"}."Write", "Error In"=w893, "Login In"=FALSE) -> ("Error Out"=w896:errorcluster)  [unwired: 6 in, 2 out]
                    n346 = Bundle By Name(cluster=w897, "Page Name"="Module - Login.vi") -> (w898:T4)
                  }
                }
              }
              frame True {
                n347 = call "Gen - Popup Single Button (Auto Close).vi"("Type"=enum16{"Error", "Info"}."Error", "Error in"=w903, "Message in"="Data acquisiton in progress.\n\nPlease stop an acquisition before logout.", "Header"="Exit") -> ("Error out"=w902:errorcluster)  [unwired: 6 in, 1 out]
              }
            }
          }
          frame "Check for Exit" {
            # "Decline exit if Data acquisition in progress."
            n348 = call "eFGV - Start Acquisition.vi"("FGV State"=State_-_eFGV."Read", "Error In"=w913) -> ("Error Out"=w911:errorcluster, "Start Out"=w909:bool)  [unwired: 7 in, 1 out]
            n349 = case shown="False" w909 {
              tunnel: w911 -> [w921 w929]
              tunnel: [w920 w928] -> w910
              tunnel: [w919 FALSE ("Yes?")] -> w908
              frame False {
                n350 = call "Gen - Popup Two Button.vi"("Type"=enum16{"Error", "Info"}."Error", "Error in"=w921, "Message in"="Are you sure to close an application?", "Header"="Exit") -> ("Error out"=w920:errorcluster, "Yes?"=w919:bool)  [unwired: 6 in]
              }
              frame True {
                n351 = call "Gen - Popup Single Button (Auto Close).vi"("Error in"=w929, "Message in"="Data acquisiton in progress.\n\nPlease stop an acquisition before exit.", "Header"="Exit") -> ("Error out"=w928:errorcluster)  [unwired: 7 in, 1 out]
              }
            }
            n352 = Select(t=State_-_Main_HMI."Close", s=w908, f=State_-_Main_HMI."Idle") -> (s? t:f=w916:T5)
          }
          frame "Close" {
            (unwired) TRUE  # Maximum?
            w951 = u8 100  # Transparency
            w952 = TRUE  # Transparently?
            n353 = call <vilib>:"Set Busy.vi"("error in (no error)"=w955) -> ("error out"=w948:errorcluster)  [unwired: 9 in, 1 out]
            n354 = call "eFGV - Stop HMI.vi"("Action"=State_-_eFGV."Write", "Error In"=w948, "Stop HMI? In"=TRUE ("Stop Main? In")) -> ("Error Out"=w947:errorcluster)  [unwired: 6 in, 2 out]
            n355 = call "Gen - SubPanel Page.vi"("State"=T9."Exit", "Error In"=w947) -> ("Error Out"=w946:errorcluster)  [unwired: 9 in]
            n356 = control-ref of="This VI"() -> (w940:refnum<vi>)
            n357 = call "Gen - VI Transparency.vi"("State"=T14."Hidden", "Error In"=w946, "Transparency"=w951, "Transparently?"=w952, "Ref VI"=w940) -> ("Error Out"=w934:errorcluster, "Ref VI Out"=w939:refnum<vi>)  [unwired: 5 in]
            n358 = call "Gen - Get Application Kind.vi"("Error In"=w934) -> ("Error Out"=w933:errorcluster, "Application:Kind"=w932:T15)  [unwired: 9 in]
            n359 = Unbundle By Name(w936) -> ("Config.HMI Configuration.HMI State"=w937:T14, "Config.HMI Configuration.Res: Width"=w931:i16, "Config.HMI Configuration.Res: Height"=w930:i16)
            n360 = case shown="\"Development System\"" w932 {
              tunnel: [w960 w967] -> w942
              tunnel: [w959 w966] -> w941
              tunnel: w939 -> [w959 w965]
              tunnel: w937 -> [_ w964]
              tunnel: w933 -> [w960 w963]
              tunnel: w931 -> [_ w962]
              tunnel: w930 -> [_ w961]
              frame "Run Time System", Default {
              }
              frame "Development System" {
                n361 = case shown="\"Standard\", Default" w964 {
                  tunnel: w963 -> [w980 w981]
                  tunnel: [w978 w981] -> w967
                  tunnel: [w975 w982] -> w966
                  tunnel: w965 -> [w973 w982]
                  tunnel: w962 -> [w969 _]
                  tunnel: w961 -> [w968 _]
                  frame "Standard", Default {
                    (unwired) i16 1356  # Width
                    (unwired) i16 655  # Height
                    # "Enable this when to set the minimum size"
                    n362 = Bundle("Res: Width"=w969, "Res: Height"=w968) -> (w972:cluster{"Res: Width":i16, "Res: Height":i16})  [unwired: 1 in]
                    n363 = Bundle("Res: Height"=w968, "Res: Width"=w969) -> (w970:cluster{"Res: Height":i16, "Res: Width":i16})  [unwired: 1 in]
                    n364 = property class="VI"(reference=w973, error in=w980, "Front Panel.Resizeable"=TRUE ("Front Panel Window:Resizable"), "Minimum Panel Size"=w972, "Front Panel.Resizeable"=FALSE ("Front Panel Window:Resizable")) -> (reference out=w976:refnum<vi>, error out=w979:errorcluster)
                    n365 = invoke class="VI" method="FP.Run-Time Position.Centered"(reference=w976, error in=w979, "Monitor"=i16 0, "Monitor"=w970) -> (reference out=w975:refnum<vi>, error out=w978:errorcluster)  [unwired: 1 in, 3 out]
                  }
                  frame "Maximized" {
                    # "Max size"
                  }
                }
              }
            }
            n366 = Unbundle By Name(w936) -> ("Event Ref"=w935:refnum<event-registration>)
            n367 = Close Reference(reference=w941, error in (no error)=w942) -> (error out=w943:errorcluster)
            n368 = call "Exit Screen.vi"("Error In"=w943) -> ("Error Out"=w944:errorcluster)  [unwired: 9 in, 1 out]
            n369 = Unregister For Events(event registration refnum=w935, error in=w944) -> (error out=w956:errorcluster)
            n370 = Wait (ms)(milliseconds to wait=u32 2000) -> ()  [unwired: 1 out]
            n371 = call <vilib>:"Unset Busy.vi"("error in (no error)"=w956) -> ("error out"=w954:errorcluster)  [unwired: 10 in]
          }
        }
      }
      frame Error {
        n372 = call <vilib>:"Clear Errors.vi"("error in (no error)"=w987) -> ("error out"=w989:errorcluster)  [unwired: 5 in, 1 out]
        n373 = call "Gen - Get Application Kind.vi"("Error In"=w989) -> ("Error Out"=w985:errorcluster, "Application:Kind"=w988:T15)  [unwired: 9 in]
        n374 = Format Into String(error in=w985, w984) -> (resulting string=w983:string)  [unwired: 2 in, 1 out]
        n375 = case shown="\"Development System\"" w988 {
          tunnel: [w994 w999 w1003] -> w986
          tunnel: w987 -> [w994 w996 w1001]
          tunnel: w983 -> [_ w995 _]
          frame "invalid app kind", Default {
          }
          frame "Run Time System" {
            n376 = control-ref of="This VI"() -> (w997:refnum<vi>)
            n377 = call "eFGV - Generated Error.vi"("eFGV States"=State_-_eFGV."Write", "Error In"=w996, "State"=w995, "This VI"=w997) -> ("Error Out"=w999:errorcluster)  [unwired: 6 in, 1 out]
          }
          frame "Development System" {
            n378 = call <vilib>:"Simple Error Handler.vi"("error in (no error)"=w1001) -> ("error?"=w1000:bool, "error out"=w1002:errorcluster)  [unwired: 4 in, 3 out]
            n379 = case shown="False" w1000 {
              tunnel: [w1004 w1006] -> w1003
              tunnel: w1002 -> [w1004 w1005]
              frame False {
              }
              frame True {
                n380 = call <vilib>:"Clear Errors.vi"("error in (no error)"=w1005) -> ("error out"=w1006:errorcluster)  [unwired: 5 in, 1 out]
              }
            }
          }
        }
        n381 = Wait (ms)(milliseconds to wait=u32 3000) -> ()  [unwired: 1 out]
      }
    }
    n382 = Wait (ms)(milliseconds to wait=u32 100) -> ()  [unwired: 1 out]
  }
  n383 = disable-structure shown="Disabled" {
    frame Disabled {
      n384 = case shown="True" {
        selector: _ -> [_ _]
        tunnel: [w1016 w1050] -> _
        tunnel: _ -> [w1017 w1051]
        tunnel: _ -> [w1011 _]
        tunnel: _ -> [w1012 w1046]
        tunnel: _ -> [w1015 w1049]
        tunnel: _ -> [w1013 w1047]
        tunnel: [T11."Enabled" ("Disabled") T11."Disabled and Grayed Out" ("Disabled")] -> _
        tunnel: [T11."Disabled and Grayed Out" ("Disabled") T11."Enabled" ("Disabled")] -> _
        tunnel: _ -> [w1009 w1044]
        tunnel: _ -> [w1008 w1043]
        tunnel: _ -> [w1007 w1042]
        frame True {
          # "Start Acquire"
          n385 = Unbundle By Name(w1007) -> ()  [unwired: 1 out]
          n386 = for {
            tunnel: w1012 -> [w1028]
            tunnel: w1011 -> [w1027] mode=indexing
            tunnel: w1015 -> [w1025]
            tunnel: w1013 -> [w1024]
            shift-right: [w1022] -> w1016
            shift-left: w1017 -> [w1026]
            tunnel: w1009 -> [w1019] mode=indexing
            tunnel: w1008 -> [w1018] mode=indexing
            n387 = case shown="True" w1024 {
              tunnel: w1025 -> [w1034 w1040]
              tunnel: w1028 -> [w1033 w1039]
              tunnel: w1027 -> [_ _]
              tunnel: [w1031 w1037] -> w1021
              tunnel: [w1030 w1036] -> w1023
              tunnel: w1026 -> [w1030 w1036]
              tunnel: w1019 -> [w1029 _]
              tunnel: w1018 -> [_ w1035]
              frame False {
                # "Stop Log"
                n388 = Search 1D Array(1D array=w1033, element=w1029) -> (index of element=w1032:i32)  [unwired: 1 in]
                n389 = Index Array(array=w1034, index=w1032) -> (element=w1031)
              }
              frame True {
                # "Start Log"
                n390 = Search 1D Array(1D array=w1039, element=w1035) -> (index of element=w1038:i32)  [unwired: 1 in]
                n391 = Index Array(array=w1040, index=w1038) -> (element=w1037)
              }
            }
            n392 = call "Gen - Button Disable.vi"("State"=enum16{"Enable", "Disable", "Disable & Gray"}."Enable", "Error In"=w1023, "Ref in"=w1021) -> ("Error Out"=w1022:errorcluster)  [unwired: 8 in]
          }
        }
        frame False {
          # "Stop Acquire"
          n393 = Unbundle By Name(w1042) -> ("Module.Enable Page"=w1041)
          n394 = for {
            tunnel: w1046 -> [w1062]
            tunnel: w1041 -> [w1061]
            tunnel: w1049 -> [w1059]
            tunnel: w1047 -> [w1058]
            shift-right: [w1056] -> w1050
            shift-left: w1051 -> [w1060]
            tunnel: w1044 -> [w1053] mode=indexing
            tunnel: w1043 -> [w1052] mode=indexing
            n395 = case shown="True" w1058 {
              tunnel: w1059 -> [w1068 w1074]
              tunnel: w1062 -> [w1067 w1073]
              tunnel: w1061 -> [w1066 w1072]
              tunnel: [w1064 w1070] -> w1055
              tunnel: [w1063 w1069] -> w1057
              tunnel: w1060 -> [w1063 w1069]
              tunnel: w1053 -> [_ _]
              tunnel: w1052 -> [_ _]
              frame False {
                # "Stop Log"
                n396 = Search 1D Array(1D array=w1067, element=w1066) -> (index of element=w1065:i32)  [unwired: 1 in]
                n397 = Index Array(array=w1068, index=w1065) -> (element=w1064)
              }
              frame True {
                # "Start Log"
                n398 = Search 1D Array(1D array=w1073, element=w1072) -> (index of element=w1071:i32)  [unwired: 1 in]
                n399 = Index Array(array=w1074, index=w1071) -> (element=w1070)
              }
            }
            n400 = call "Gen - Button Disable.vi"("State"=enum16{"Enable", "Disable", "Disable & Gray"}."Enable", "Error In"=w1057, "Ref in"=w1055) -> ("Error Out"=w1056:errorcluster)  [unwired: 8 in]
          }
        }
      }
    }
    frame Enabled {
    }
  }
  n401 = call "Main - Init Close Variable.vi"("State"=enum16{"Init", "Close"}."Close", "Error In"=w15) -> ("Error Out"=w14:errorcluster)  [unwired: 9 in]
  n402 = control-ref of="This VI"() -> (w12:refnum<vi>)
  n403 = call "Gen - Close VI.vi"("Error In"=w14, "Ref VI"=w12) -> ("Error Out"=→"Error out":errorcluster)  [unwired: 9 in]
